vi "Comparing Different Hierarchical Linkage.vi"() -> ()   [LabVIEW 2020]
doc: "This example shows characteristics of different linkage methods for hierarchical clustering on datasets that are “interesting” but still in 2D.\n\nThe main observations to make are :\n\n - single linkage is fast, and can perform well on non-globular data, but it performs poorly in the presence of noise.\n\n- average and complete linkage perform well on cleanly separated globular clusters, but have mixed results otherwise.\n\n- Ward is the most effective method for noisy data.\n\nWhile these examples give some intuition about the algorithms, this intuition might not apply to very high dimensional data."
uses:
  Model/Unsupervised/Cluster/AgglomerativeClustering/controls/agglomerative_clustering_params.ctl
  PLAIYDISPLAY/Display/Classification/2D/Predicted/Controls/PredictedParameter.ctl
  PLAIYDISPLAY/Display/_Controls/Style.ctl
  <vilib>/Analysis/baseanly.llb/Real A x B.vi
  Model/Unsupervised/Cluster/AgglomerativeClustering/AgglomerativeClustering.lvclass
  C:/Users/cipop/TDF Dropbox/2_Technologies de France/1 - Services et Etudes/PLAIY/2 - DEV/PLAIYLAB/code/Model/Model.lvclass
  Preproc/Objet/6 - Datasets Transformation/6.3 - Processing Data/StandardScaler/StandardScaler.vi
  Model/Unsupervised/Cluster/AgglomerativeClustering/AgglomerativeClustering.vi
  <vilib>/Analysis/Matrix/Numeric/Conversions/Array To Matrix - RA2.vi
  <vilib>/Analysis/Matrix/Numeric/Conversions/Matrix To Array - RM.vi
  Preproc/Objet/6 - Datasets Transformation/6.3 - Processing Data/StandardScaler/StandardScaler.lvclass
  <vilib>/Analysis/Matrix/NI_Matrix.lvlib
  <vilib>/Analysis/NI_AALBase.lvlib
panel:
  out "X_aniso":dbl[][](array[numeric])
  in  "error in":errorcluster
  out "error out":errorcluster
  out "Plot 24":cluster{"X":dbl[], "Y":dbl[]}[](graph) caption="Ward Linkage"
  out "no_structure":dbl[][](array[numeric])
  out "Plot 23":cluster{"X":dbl[], "Y":dbl[]}[](graph) caption="Complete Linkage"
  out "Plot 22":cluster{"X":dbl[], "Y":dbl[]}[](graph) caption="Average Linkage"
  out "Plot 21":cluster{"X":dbl[], "Y":dbl[]}[](graph) caption="Single Linkage"
  out "Plot 20":cluster{"X":dbl[], "Y":dbl[]}[](graph) caption="Ward Linkage"
  out "varied":dbl[][](array[numeric])
  out "Plot 19":cluster{"X":dbl[], "Y":dbl[]}[](graph) caption="Complete Linkage"
  out "Plot 18":cluster{"X":dbl[], "Y":dbl[]}[](graph) caption="Average Linkage"
  out "Plot 17":cluster{"X":dbl[], "Y":dbl[]}[](graph) caption="Single Linkage"
  out "Plot 16":cluster{"X":dbl[], "Y":dbl[]}[](graph) caption="Ward Linkage"
  out "aniso":dbl[][](array[numeric])
  out "Plot 15":cluster{"X":dbl[], "Y":dbl[]}[](graph) caption="Complete Linkage"
  out "Plot 14":cluster{"X":dbl[], "Y":dbl[]}[](graph) caption="Average Linkage"
  out "Plot 13":cluster{"X":dbl[], "Y":dbl[]}[](graph) caption="Single Linkage"
  out "Plot 12":cluster{"X":dbl[], "Y":dbl[]}[](graph) caption="Ward Linkage"
  out "blobs":dbl[][](array[numeric])
  out "Plot 11":cluster{"X":dbl[], "Y":dbl[]}[](graph) caption="Complete Linkage"
  out "Plot 10":cluster{"X":dbl[], "Y":dbl[]}[](graph) caption="Average Linkage"
  out "Plot 9":cluster{"X":dbl[], "Y":dbl[]}[](graph) caption="Single Linkage"
  out "Plot 8":cluster{"X":dbl[], "Y":dbl[]}[](graph) caption="Ward Linkage"
  out "noisy_moons":dbl[][](array[numeric])
  out "Plot 7":cluster{"X":dbl[], "Y":dbl[]}[](graph) caption="Complete Linkage"
  out "Plot 6":cluster{"X":dbl[], "Y":dbl[]}[](graph) caption="Average Linkage"
  out "Plot 5":cluster{"X":dbl[], "Y":dbl[]}[](graph) caption="Single Linkage"
  out "Plot 4":cluster{"X":dbl[], "Y":dbl[]}[](graph) caption="Single Linkage"
  out "Plot 3":cluster{"X":dbl[], "Y":dbl[]}[](graph) caption="Average Linkage"
  out "Plot 2":cluster{"X":dbl[], "Y":dbl[]}[](graph) caption="Complete Linkage"
  out "noisy_circles":dbl[][](array[numeric])
  out "Plot":cluster{"X":dbl[], "Y":dbl[]}[](graph) caption="Ward Linkage"
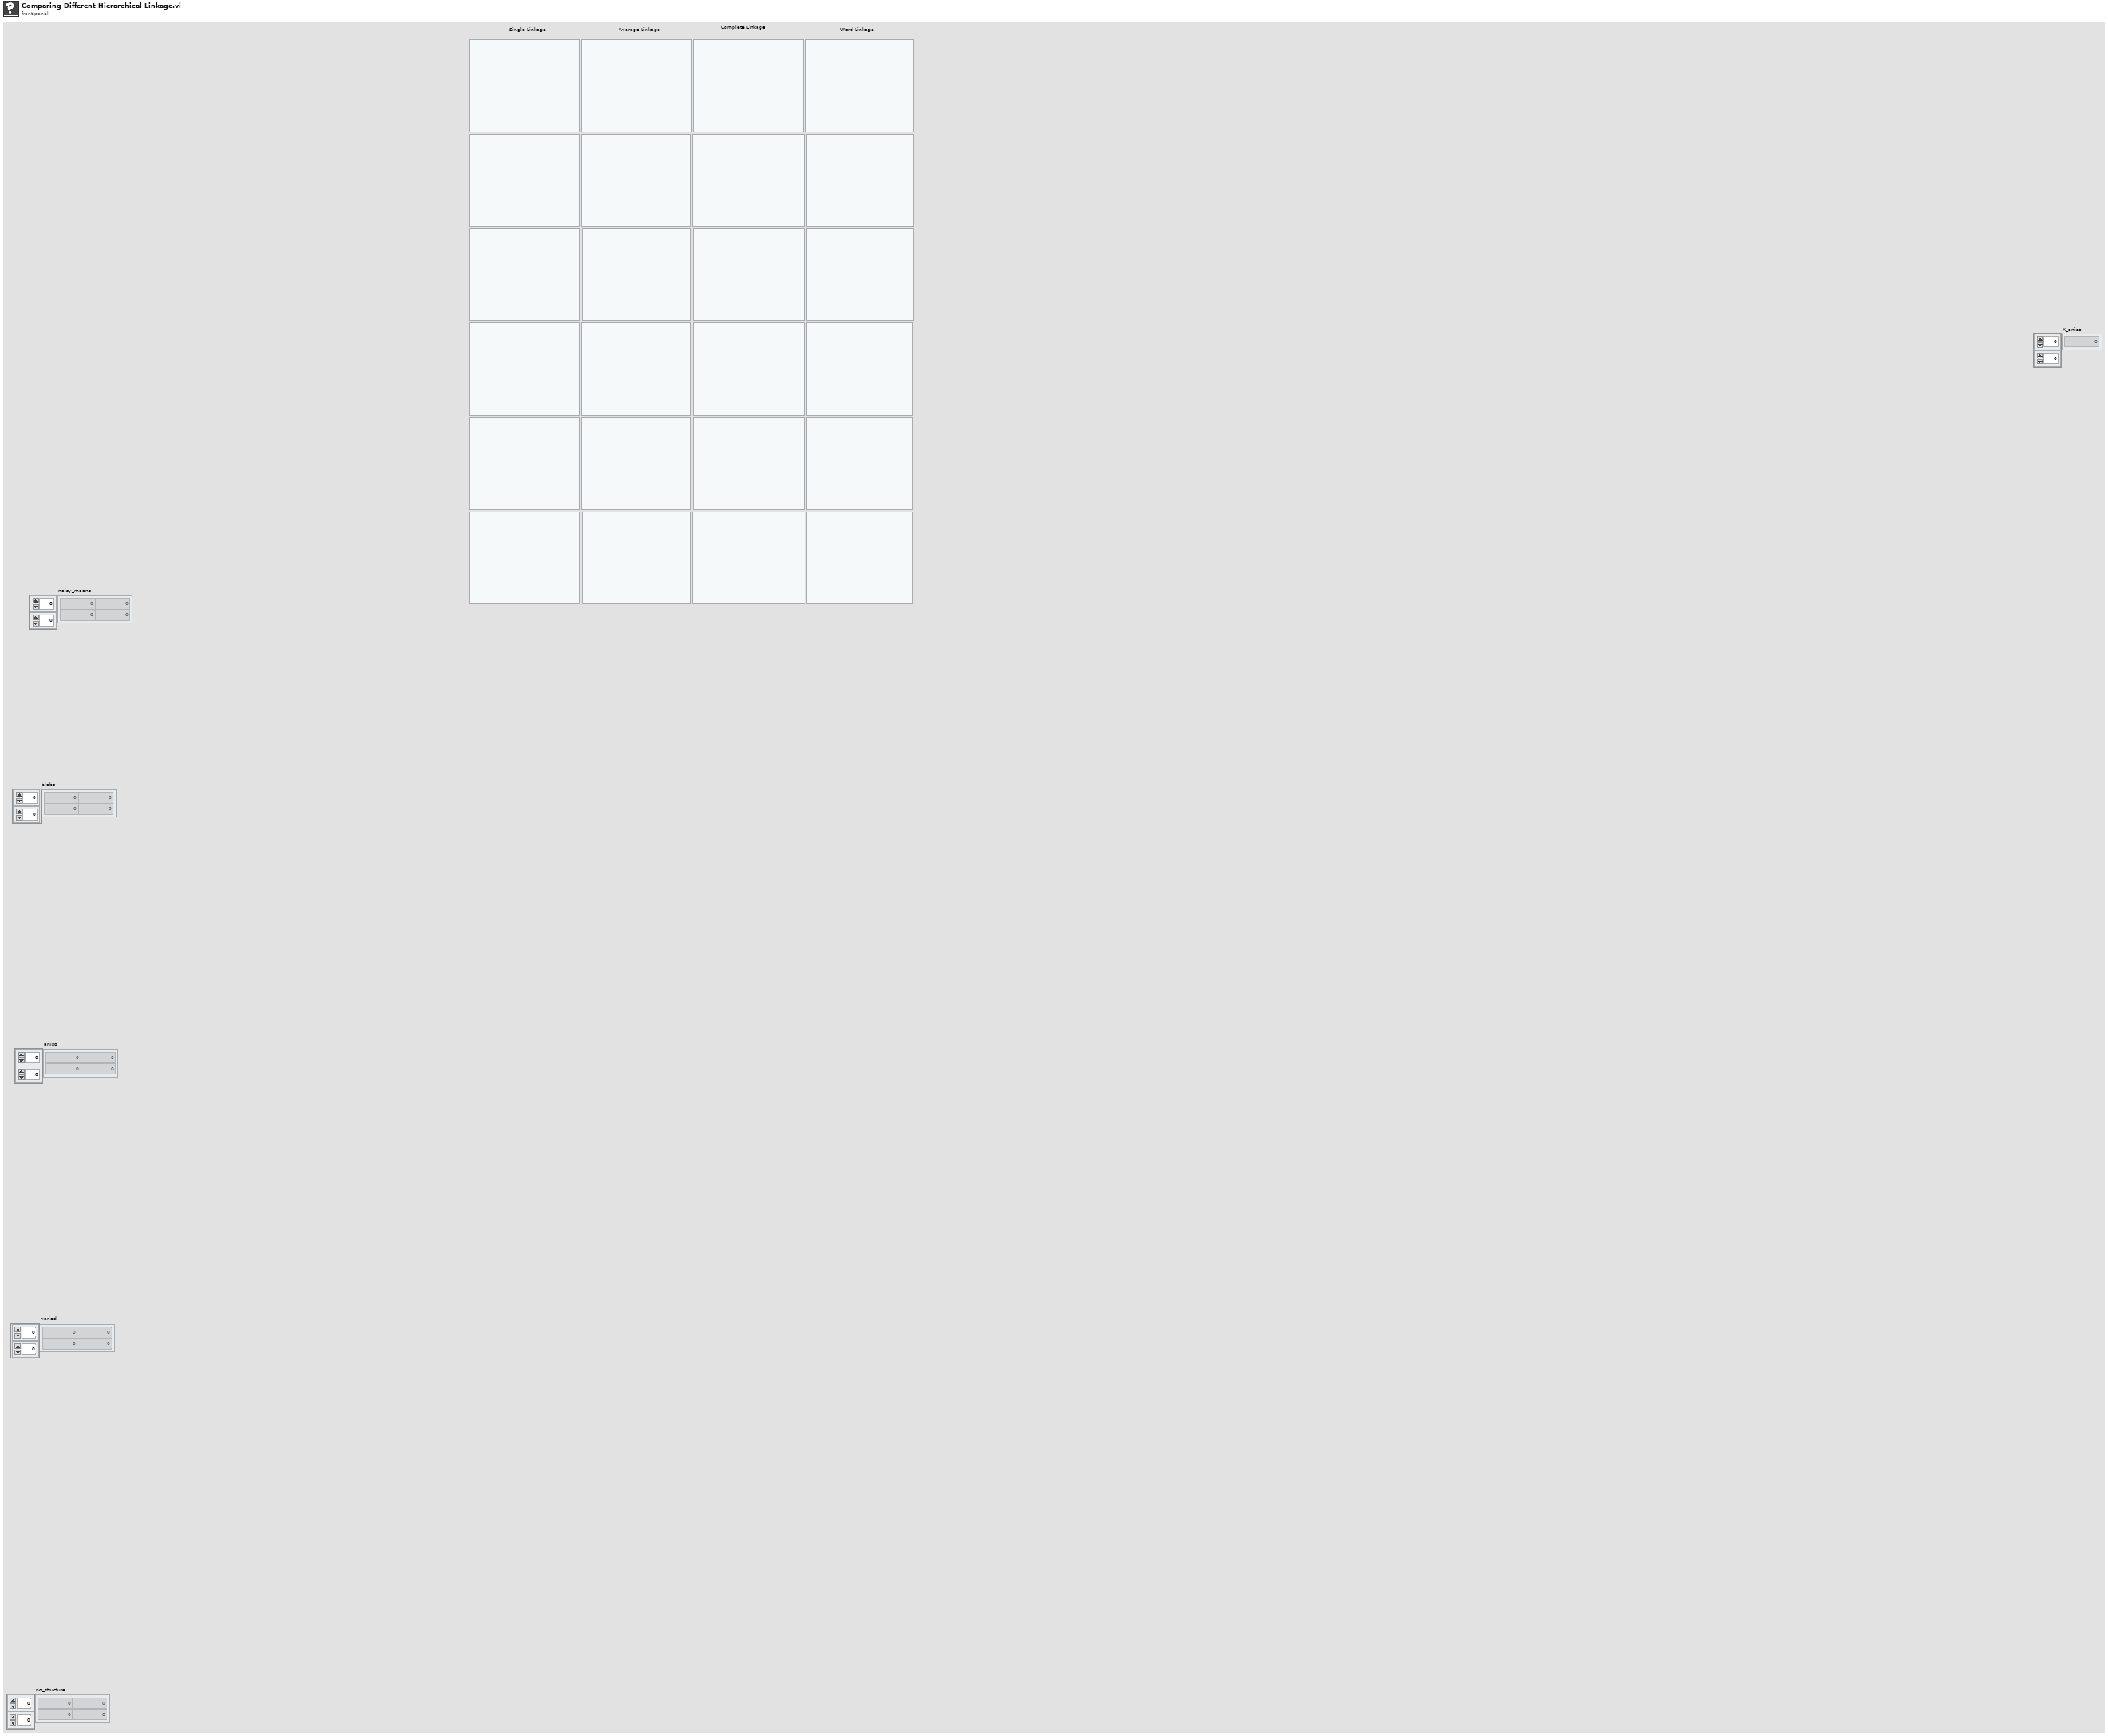
[diagram p1: front panel]
types:
  T1 = enum16{"Numeric Array", "String Array", "Sparse"}
  T2 = cluster{"n_samples":string, "shuffle":bool, "noise":dbl, "random_state":i32, "factor":dbl, "Returns":string}
  T3 = typedef "Style.ctl" = enum16{"Empty circle", "Full circle", "Empty square", "Full square", "Cross"}
  T4 = typedef "PredictedParameter.ctl" = cluster{"Plot":refnum<vi>, "Data":cluster{"X":dbl[][], "Predict":dbl[][]}, "Indexe":cluster{"X":i32, "Y":i32}, "Point Property":cluster{"Style":T3, "Label Color":u32[]}}
  T5 = typedef "agglomerative_clustering_params.ctl" = cluster{"n_clusters":cluster{"n_clusters_type":string, "n_clusters_int":dbl}, "affinity":cluster{"affinity_type":string, "affinity_function":string}, "memory":string, "connectivity":cluster{"connectivity_type":string, "connectivity_list":dbl[][]}, "compute_full_tree":cluster{"compute_full_tree_type":string, "compute_full_tree_bool":bool}, "linkage":string, "distance_threshold":cluster{"distance_threshold_type":string, "distance_threshold_float":dbl}, "compute_distances":bool}
  T6 = cluster{"n_clusters_type":string, "n_clusters_int":dbl}
  T7 = cluster{"n_samples":string, "shuffle":bool, "noise":dbl, "random_state":i32, "Returns":string}
  T8 = cluster{"n_samples":i32[], "n_features":u32, "centers":i32[][], "cluster_std":dbl[], "centermin":dbl, "centermax":dbl, "shuffle":bool, "random_state":i32, "Returns":string}
  T9 = cluster{" 4DArray":cluster{"1":string[][], "2":string[][]}[], " 3DArray":cluster{"Tableau":string[][]}[], "Sparse Matrix 2DArray":string[][], " 2DArray":string[][], " 1DArray":string[]}
  T10 = typedef "agglomerative_clustering_attributes.ctl" = cluster{"n_clusters_":dbl, "labels_":dbl[], "n_leaves_":dbl, "n_connected_components_":dbl, "children_":dbl[][], "distances_":dbl[]}
  T11 = typedef "NI_Matrix.lvlib/RealMatrix.ctl" = dbl[][]
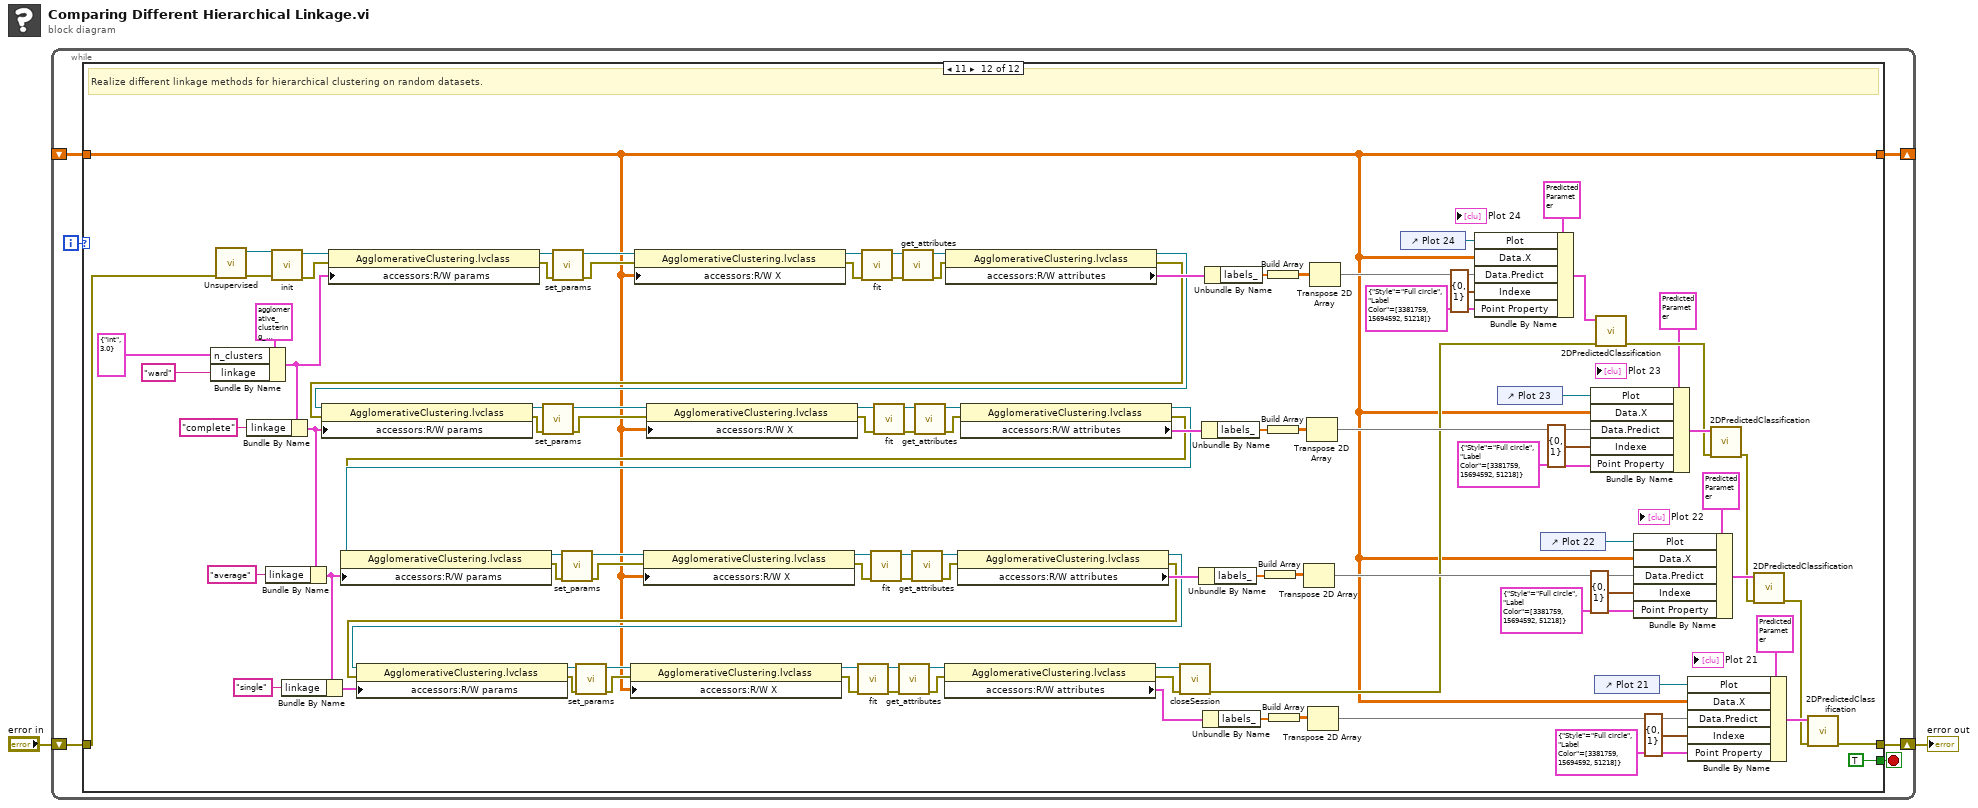
[diagram p0: block diagram]
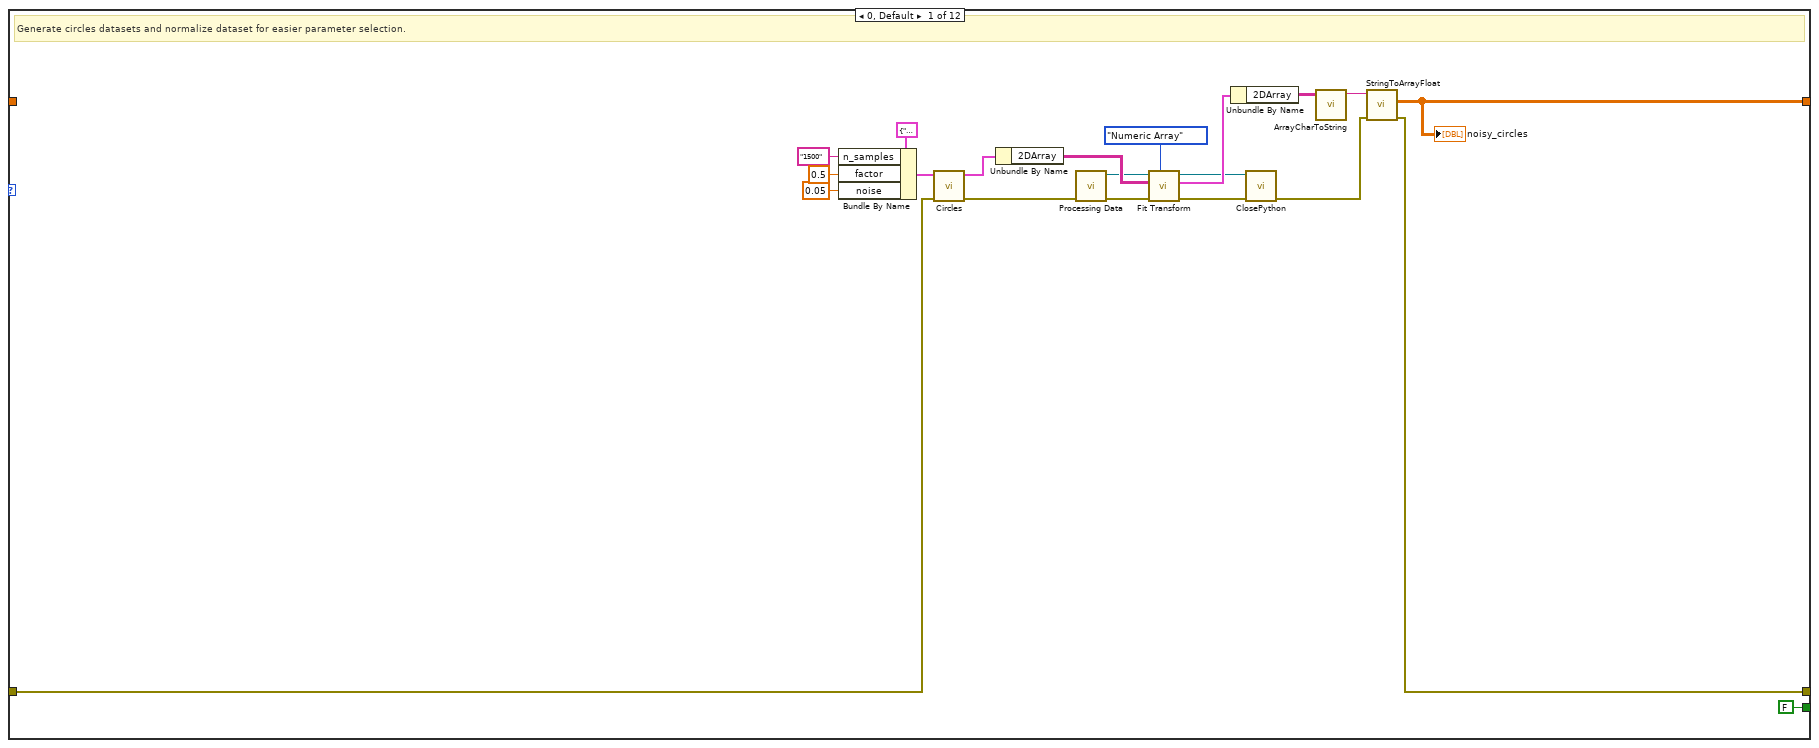
[diagram p2: hidden frame]
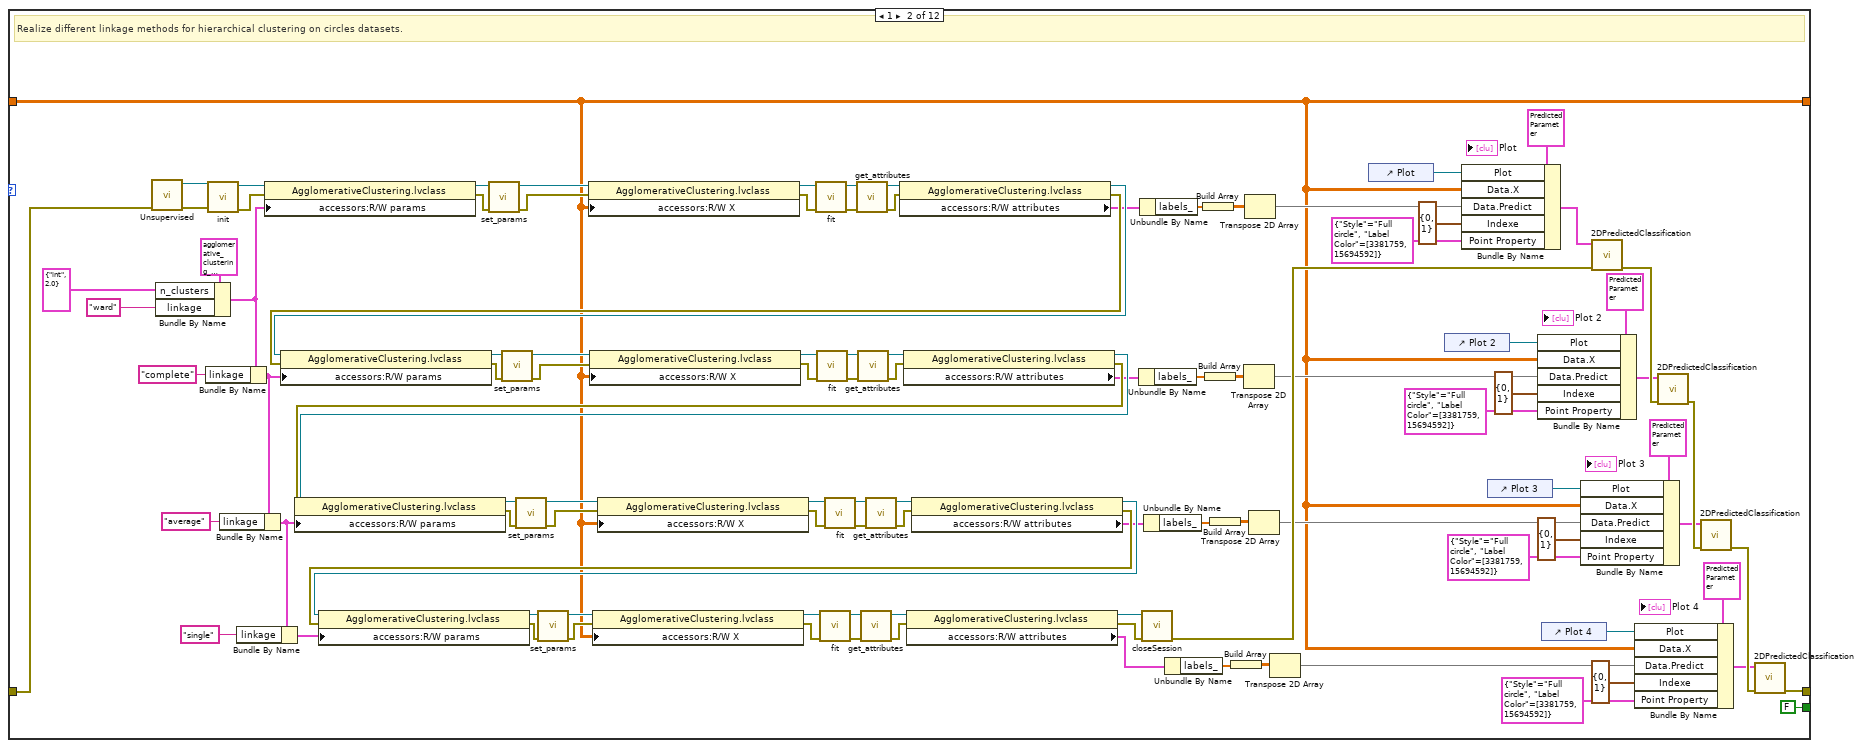
[diagram p3: hidden frame]
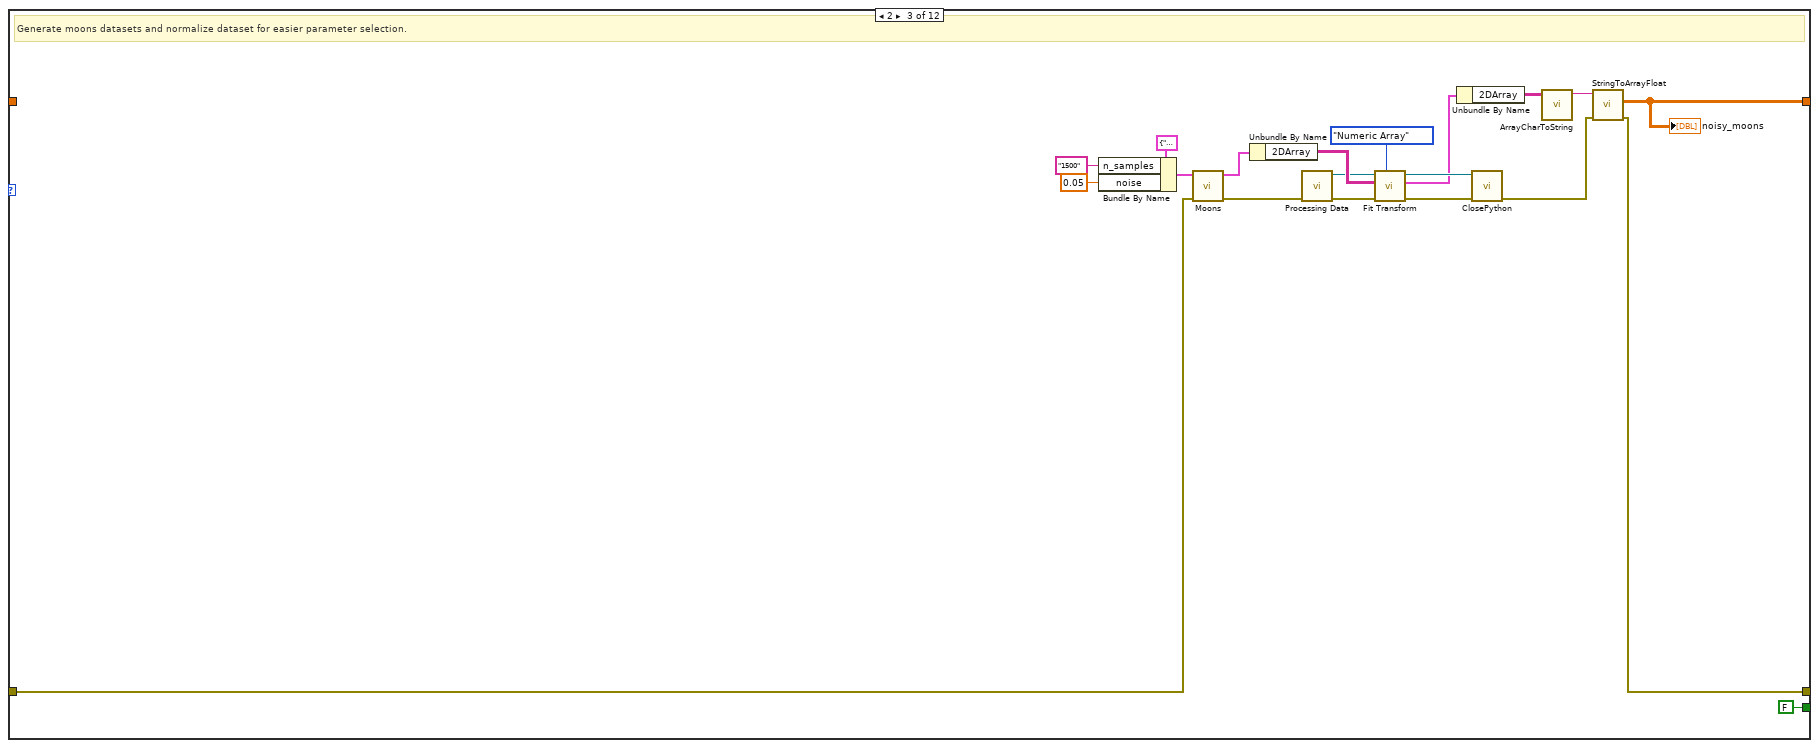
[diagram p4: hidden frame]
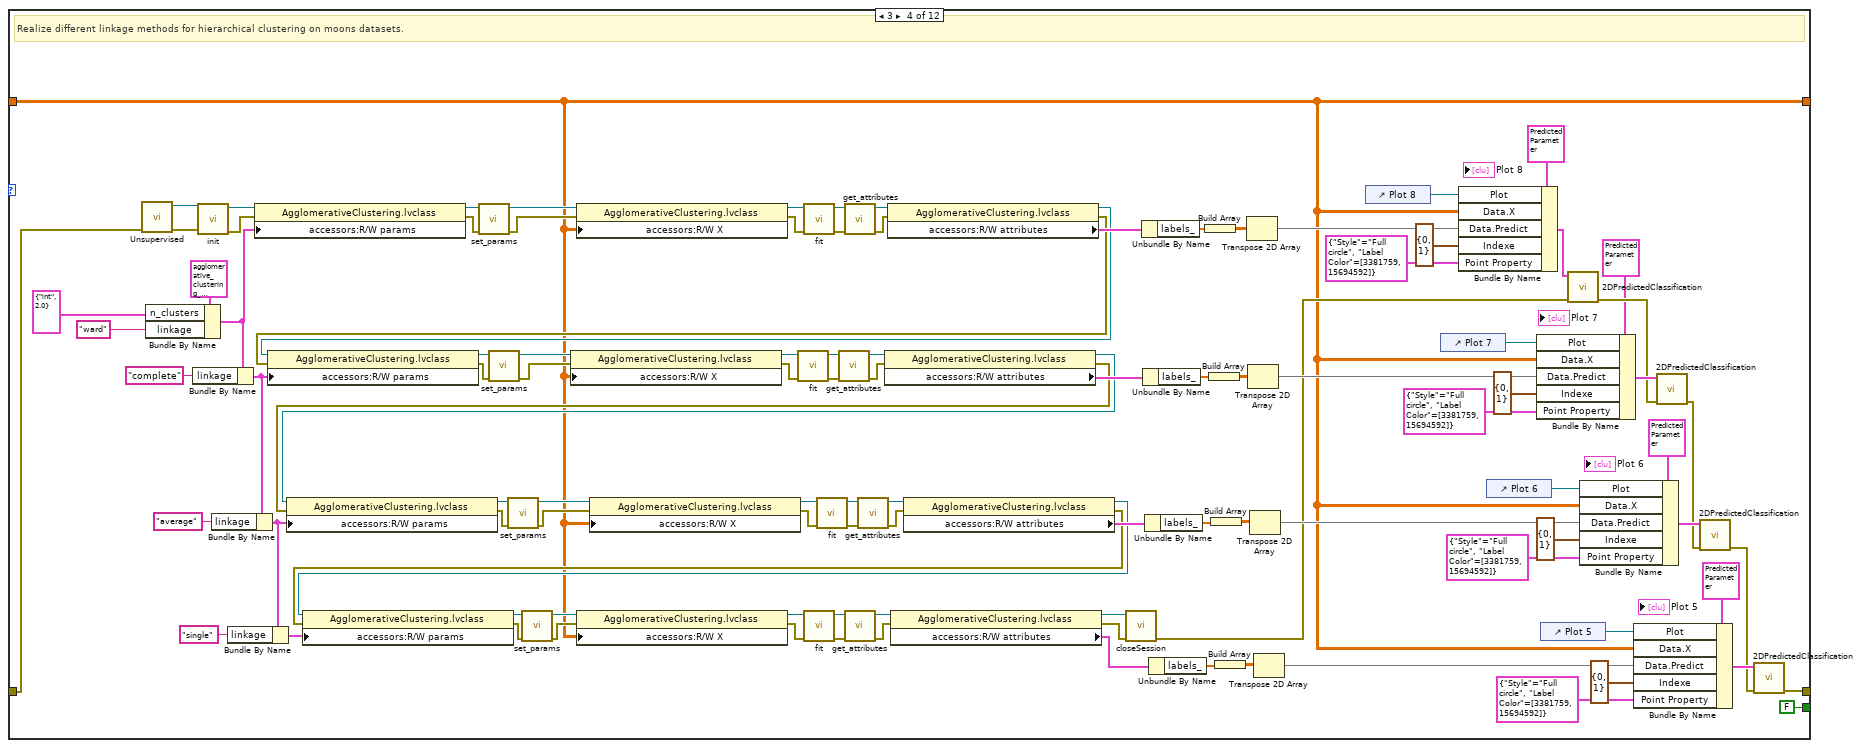
[diagram p5: hidden frame]
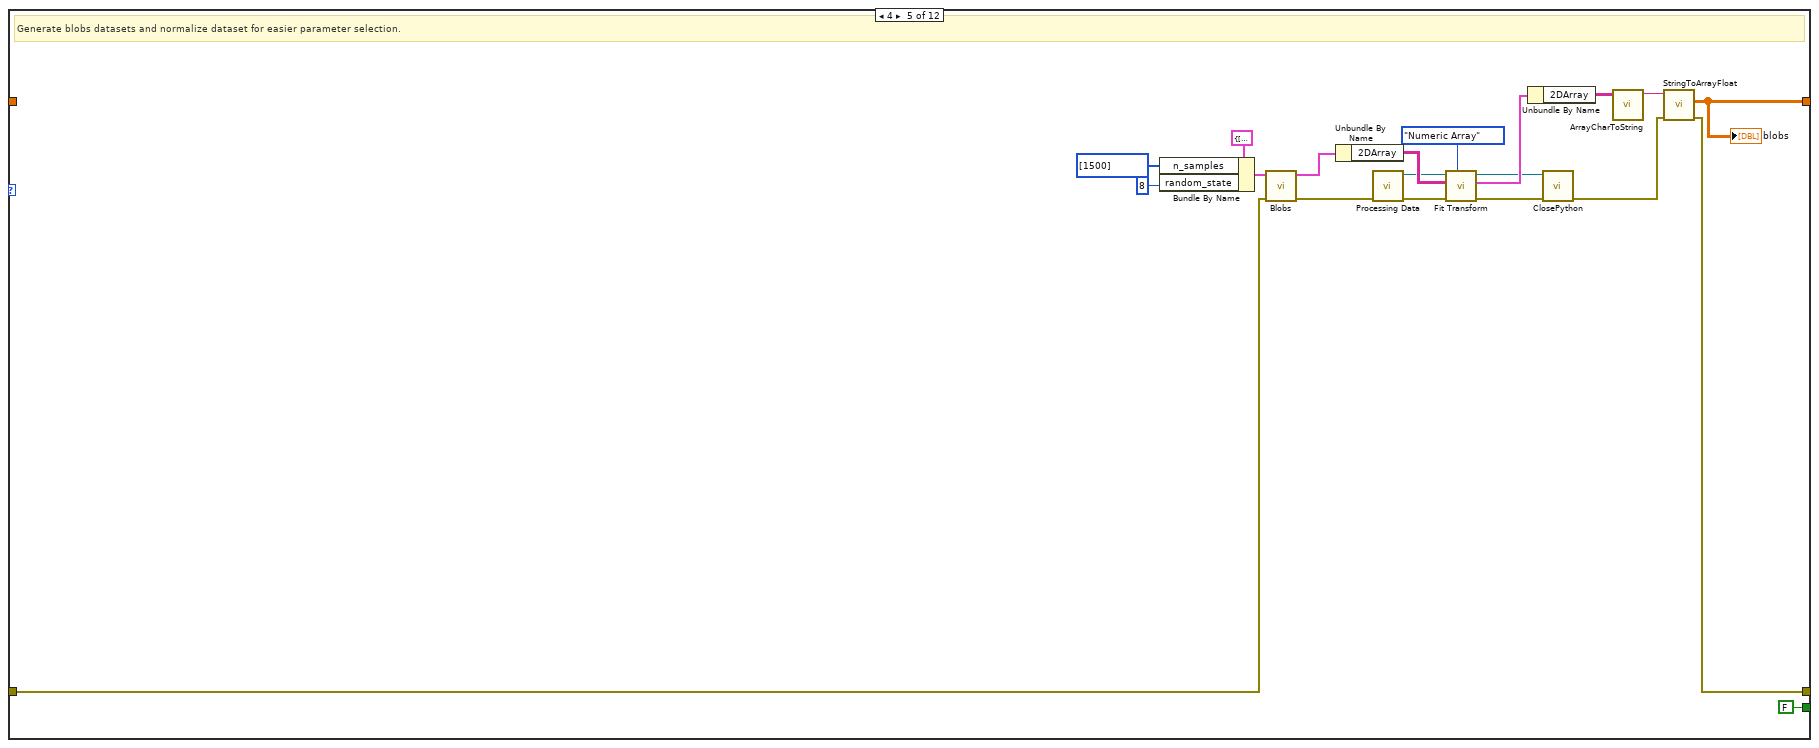
[diagram p6: hidden frame]
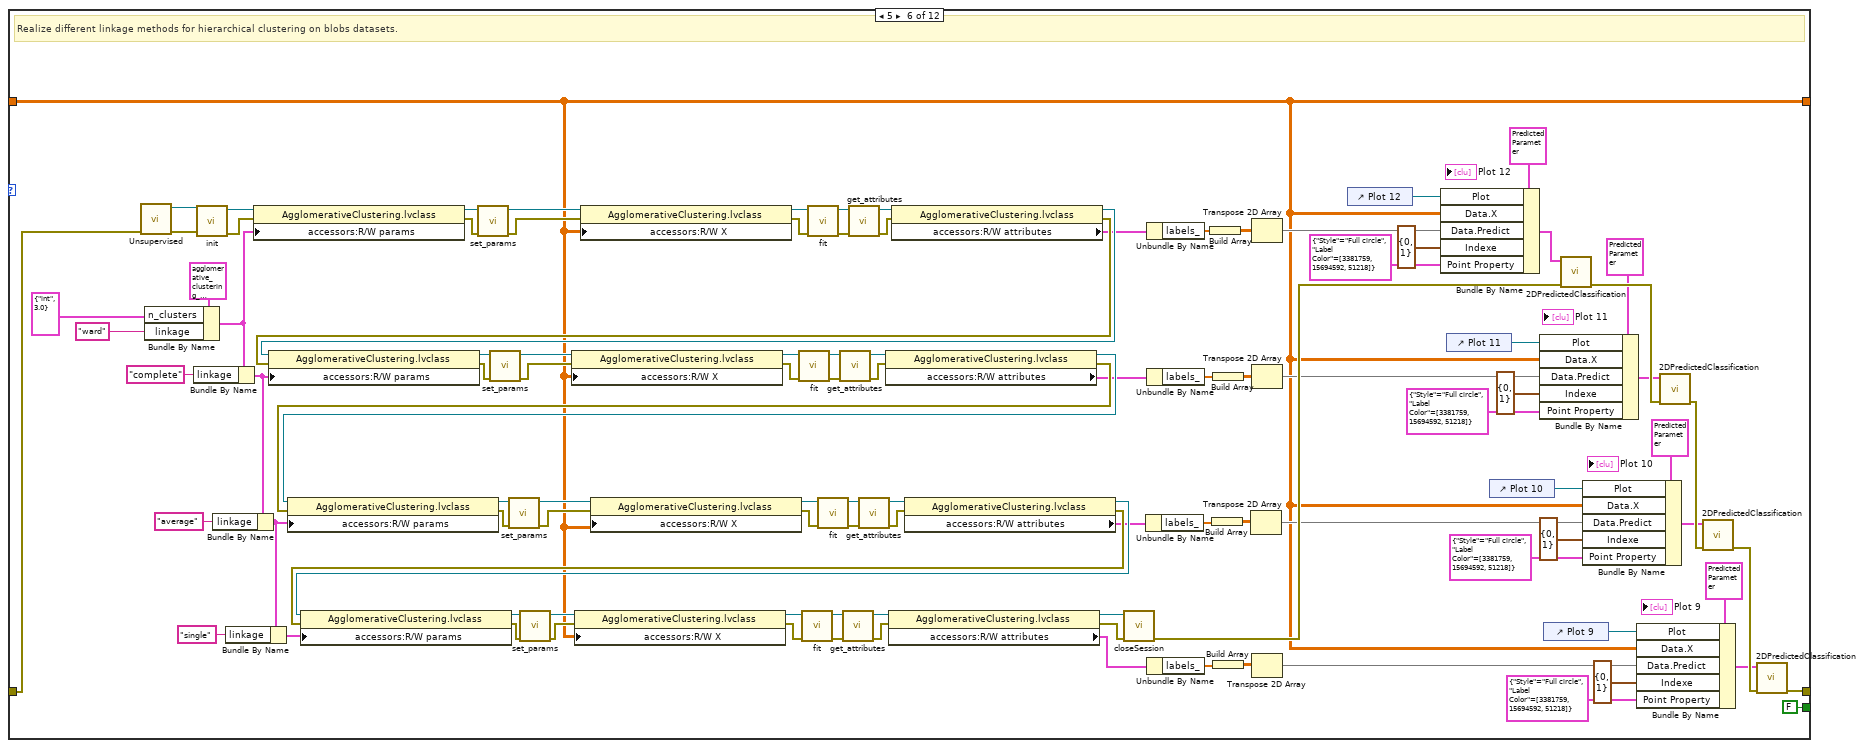
[diagram p7: hidden frame]
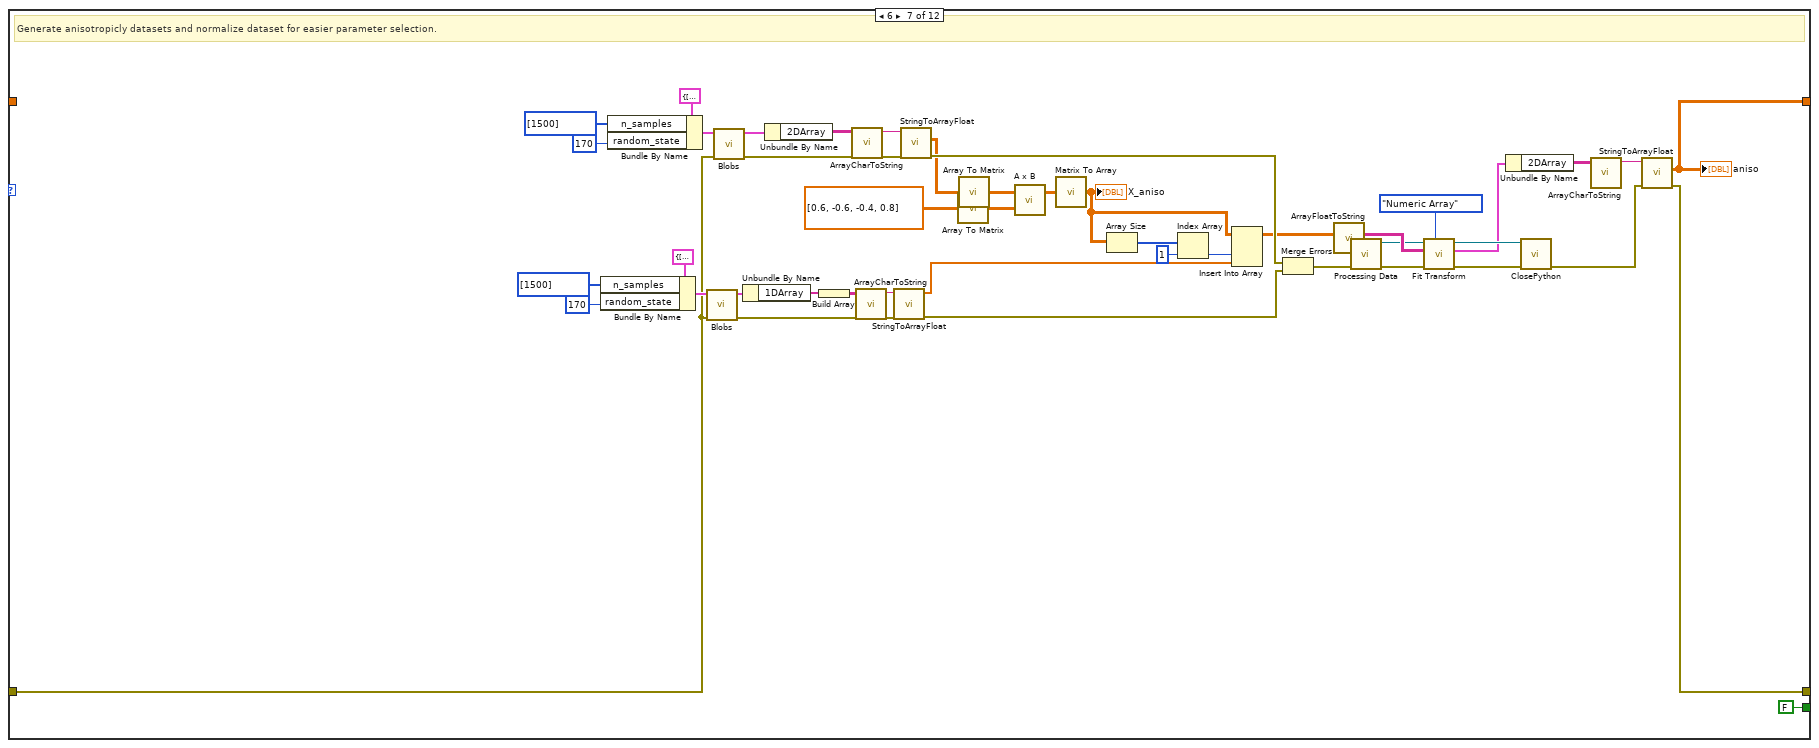
[diagram p8: hidden frame]
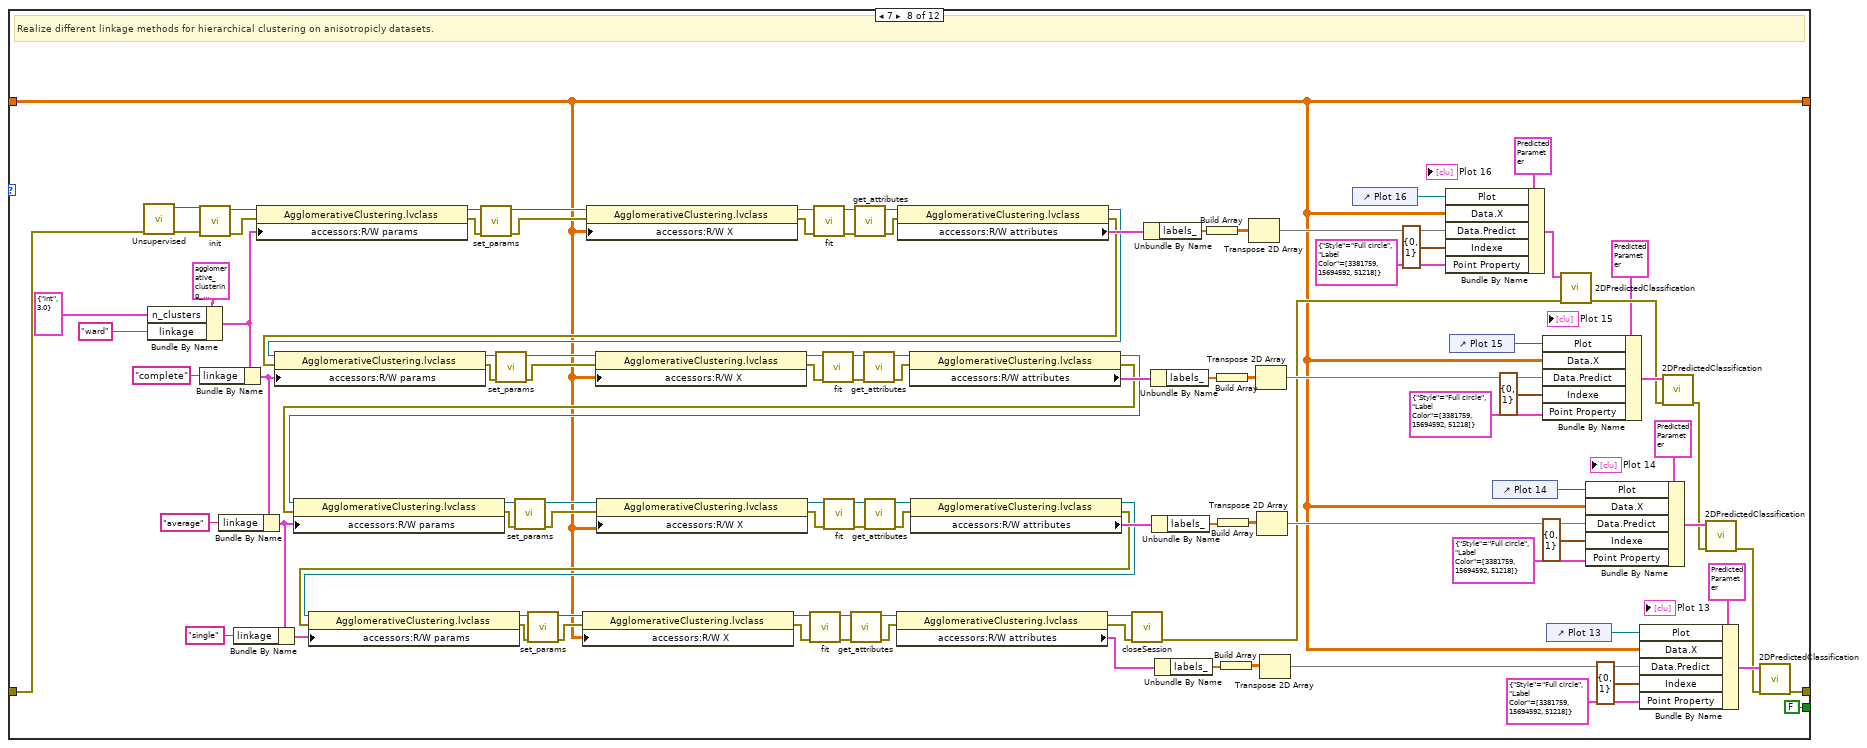
[diagram p9: hidden frame]
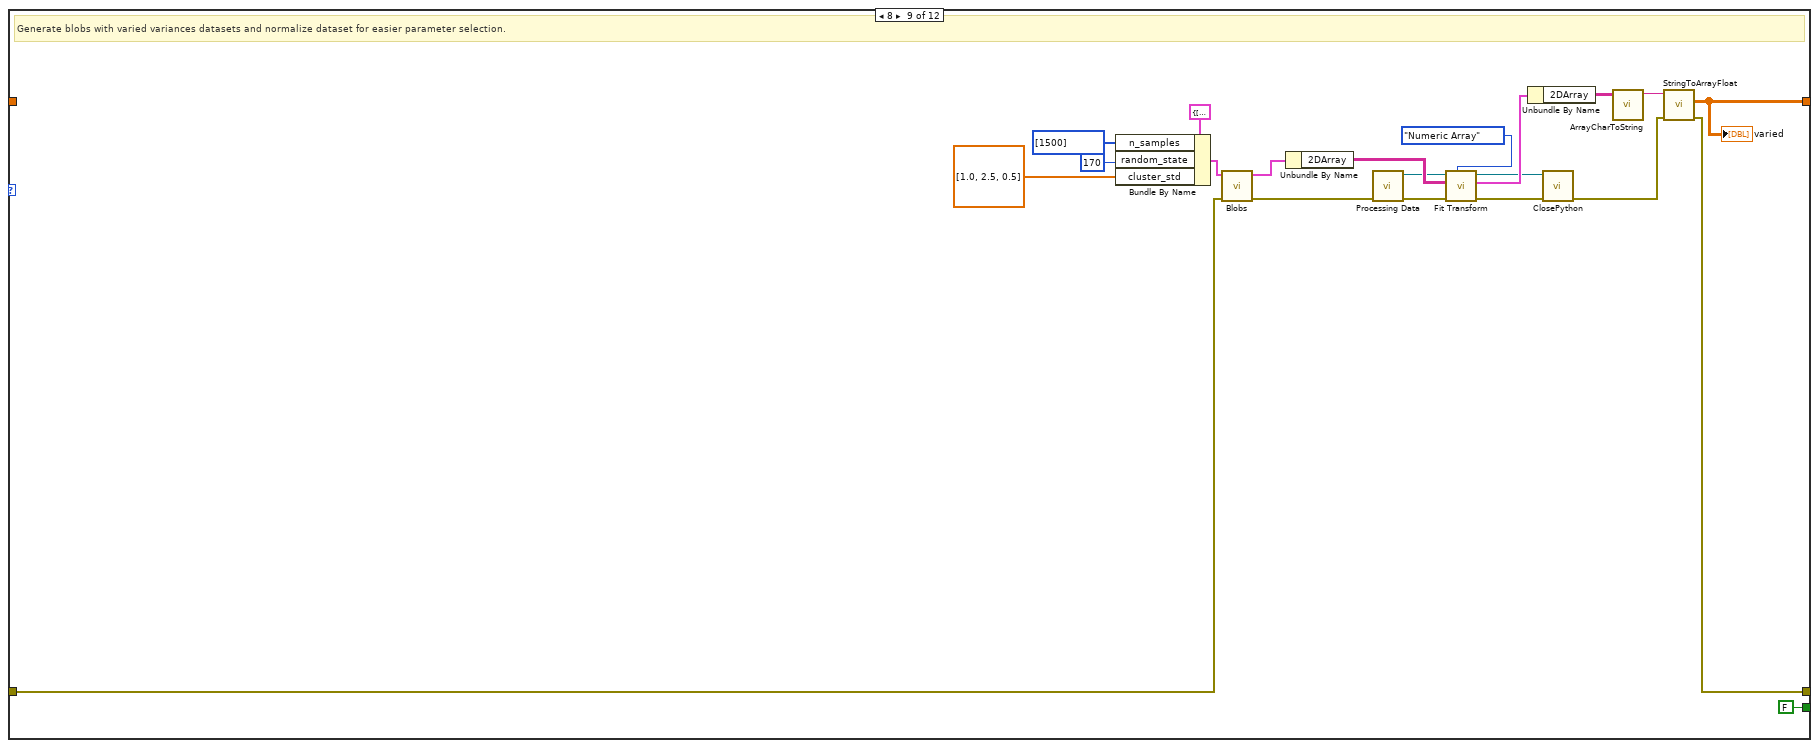
[diagram p10: hidden frame]
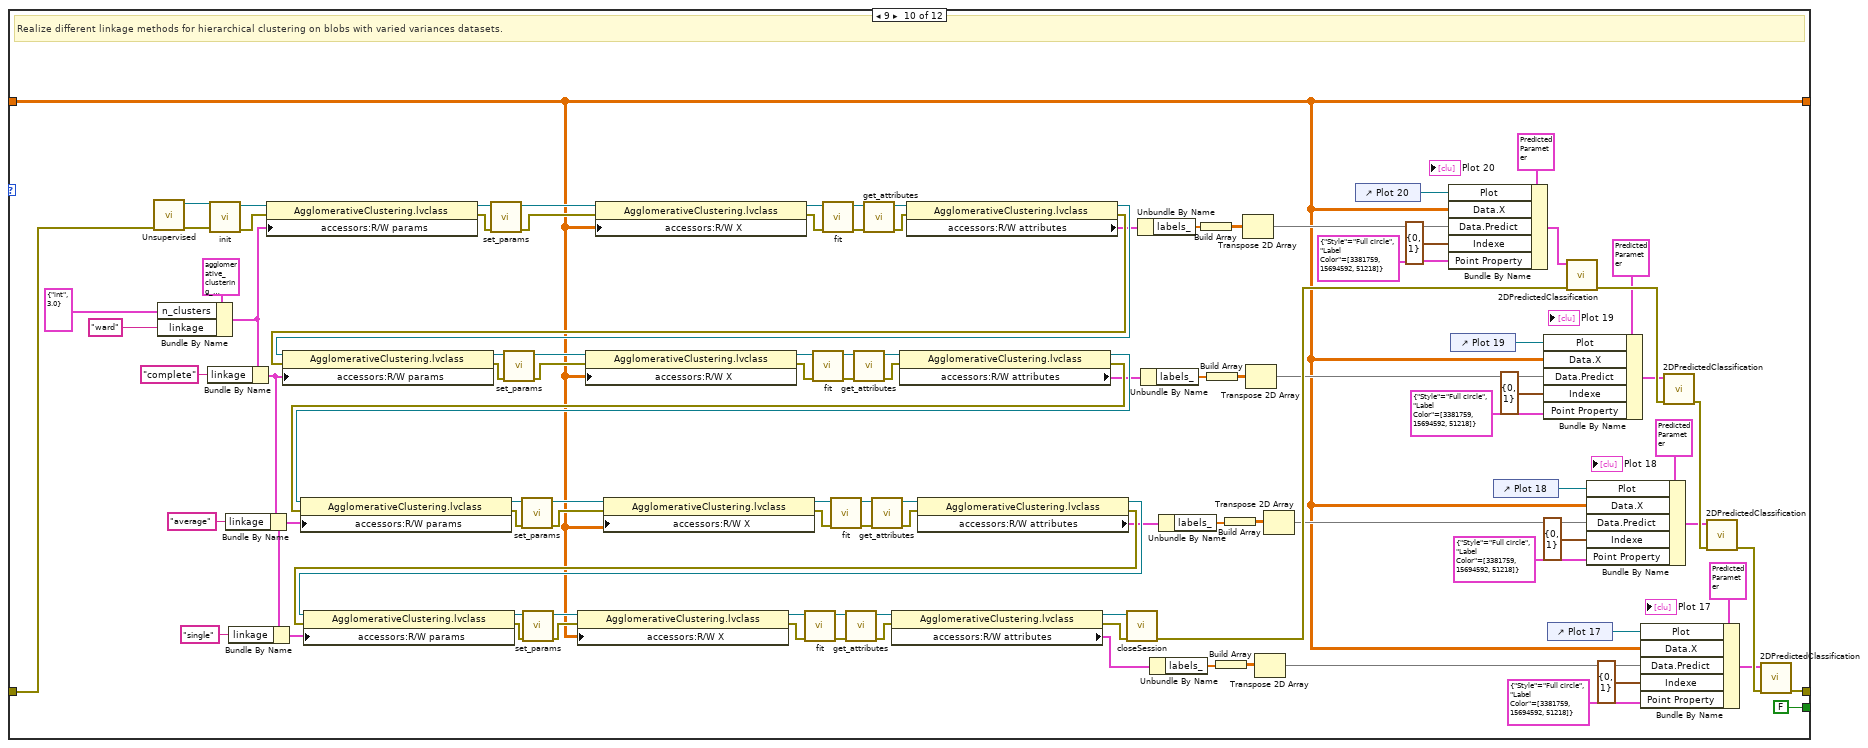
[diagram p11: hidden frame]
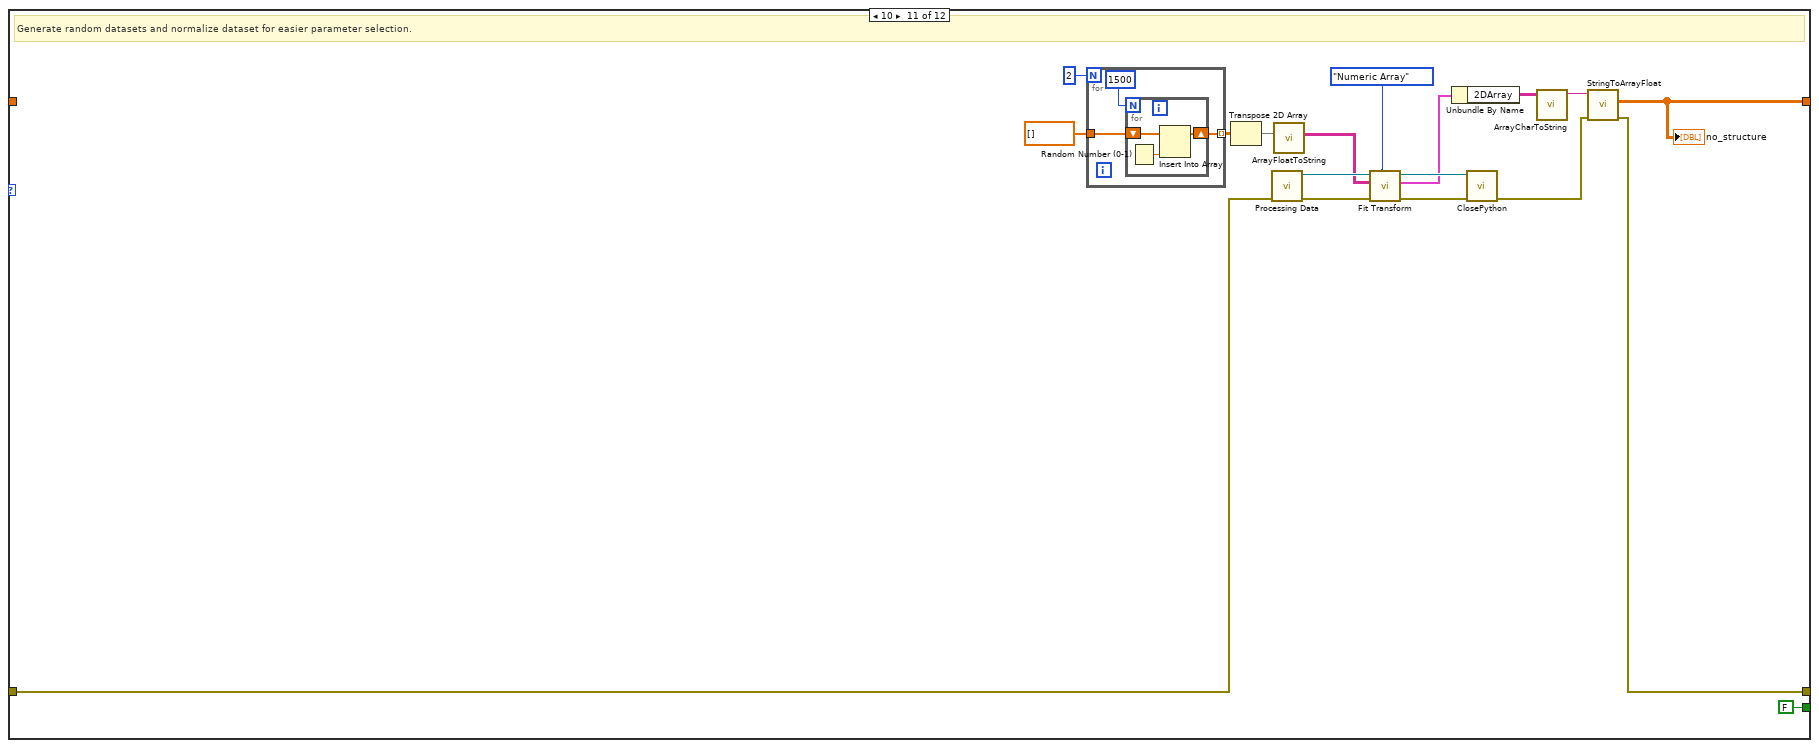
[diagram p12: hidden frame]
diagram:
  n1 = while {
    shift-right: [w5] -> w1
    shift-left: "error in" -> [w6]
    shift-right: [w4] -> _
    shift-left: _ -> [w3]
    i -> [w8]
    stop <- w7 stop-if-true
    n2 = case shown="11" w8 {
      tunnel: [FALSE FALSE FALSE FALSE FALSE FALSE FALSE FALSE FALSE FALSE FALSE TRUE] -> w7
      tunnel: w6 -> [w12 w31 w137 w157 w263 w283 w391 w434 w540 w561 w667 w691]
      tunnel: [w10 w32 w139 w162 w265 w288 w390 w435 w542 w562 w669 w693] -> w5
      tunnel: [w11 w30 w136 w156 w262 w282 w388 w433 w539 w560 w666 w690] -> w4
      tunnel: w3 -> [_ w30 _ w156 _ w282 _ w433 _ w560 _ w690]
      frame 0, Default {
        # "Generate circles datasets and normalize dataset for easier parameter selection."
        n3 = Bundle By Name(cluster=T2 {"n_samples"="100", "shuffle"=TRUE, "noise"=-1.0, "random_state"=-1, "factor"=0.8, "Returns"="X"} ("make_circles"), "n_samples"="1500", "factor"=0.5, "noise"=0.05) -> (w19:T2)
        n4 = call "Circles.vi"("error in (no error)"=w12, "make_circles"=w19) -> ("error out"=w26:errorcluster, "Data"=w18:T9)  [unwired: 8 in]
        n5 = Unbundle By Name(w18) -> ("2DArray"=w24:string[][])
        n6 = call-poly "Processing Data.vi"("error in (no error)"=w26) -> ("error out"=w21:errorcluster, "StandardScaler.lvclass"=w20:refnum<class "StandardScaler.lvclass">)  [unwired: 9 in]
        n7 = call-dynamic "Fit Transform.vi"("Type X"=T1."Numeric Array", "error in (no error)"=w21, "X"=w24, "StandardScaler.lvclass"=w20) -> ("error out"=w23:errorcluster, "Data"=w25:T9, "StandardScaler.lvclass"=w22:refnum<class "StandardScaler.lvclass">)  [unwired: 5 in]
        n8 = Unbundle By Name(w25) -> ("2DArray"=w28:string[][])
        n9 = call-dynamic "ClosePython.vi"("error in (no error)"=w23, "Scikit-learn en entrée"=w22) -> ("error out"=w29:errorcluster)  [unwired: 8 in, 1 out]
        n10 = call "ArrayCharToString.vi"("TAB"=w28) -> ("Instruction"=w27:string)  [unwired: 10 in]
        n11 = call "StringToArrayFloat.vi"("entrée d'erreur (pas d'erreur)"=w29, "Return value"=w27) -> ("error IO"=w10:errorcluster, "2DArray"=w11:dbl[][])  [unwired: 7 in, 1 out]
        "noisy_circles" <- w11
      }
      frame 1 {
        # "Realize different linkage methods for hierarchical clustering on circles datasets."
        n12 = call-poly "Unsupervised.vi"("error in"=w31) -> ("error out"=w57:errorcluster, "out"=w56:refnum<class "AgglomerativeClustering.lvclass">)  [unwired: 9 in]
        n13 = Bundle By Name(cluster=T5 {"n_clusters"={"n_clusters_type"="int", "n_clusters_int"=0.0}, "affinity"={"affinity_type"="euclidean", "affinity_function"="metric_function"}, "memory"="", "connectivity"={"connectivity_type"="None", "connectivity_list"=[]}, "compute_full_tree"={"compute_full_tree_type"="auto", "compute_full_tree_bool"=FALSE}, "linkage"="ward", "distance_threshold"={"distance_threshold_type"="None", "distance_threshold_float"=0.0}, "compute_distances"=FALSE} ("output cluster"), "n_clusters"=T6 {"n_clusters_type"="int", "n_clusters_int"=2.0}, "linkage"="ward") -> (w81:T5)
        n14 = Bundle By Name(cluster=w81, "linkage"="complete") -> (w96:T5)
        n15 = call-dynamic "init.vi"("error in (no error)"=w57, "Model en entrée"=w56) -> ("error out"=w58:errorcluster, "Model en sortie"=w52:refnum<class "AgglomerativeClustering.lvclass">)  [unwired: 8 in]
        n16 = Bundle By Name(cluster=w96, "linkage"="average") -> (w114:T5)
        n17 = Bundle By Name(cluster=w114, "linkage"="single") -> (w112:T5)
        n18 = property class="AgglomerativeClustering.lvclass"(reference=w52, error in=w58, "accessors:R/W params"=w81) -> (reference out=w53:refnum<class "AgglomerativeClustering.lvclass">, error out=w59:errorcluster)
        n19 = call-dynamic "set_params.vi"("error in (no error)"=w59, "AgglomerativeClustering.lvclass 2"=w53) -> ("error out"=w60:errorcluster, "AgglomerativeClustering.lvclass"=w54:refnum<class "AgglomerativeClustering.lvclass">)  [unwired: 8 in]
        n20 = property class="AgglomerativeClustering.lvclass"(reference=w54, error in=w60, "accessors:R/W X"=w30) -> (reference out=w51:refnum<class "AgglomerativeClustering.lvclass">, error out=w61:errorcluster)
        n21 = call-dynamic "fit.vi"("error in (no error)"=w61, "AgglomerativeClustering.lvclass 2"=w51) -> ("error out"=w62:errorcluster, "AgglomerativeClustering.lvclass"=w55:refnum<class "AgglomerativeClustering.lvclass">)  [unwired: 8 in]
        n22 = call-dynamic "get_attributes.vi"("error in (no error)"=w62, "AgglomerativeClustering.lvclass 2"=w55) -> ("error out"=w68:errorcluster, "AgglomerativeClustering.lvclass"=w67:refnum<class "AgglomerativeClustering.lvclass">)  [unwired: 8 in]
        n23 = property class="AgglomerativeClustering.lvclass"(reference=w67, error in=w68) -> (reference out=w82:refnum<class "AgglomerativeClustering.lvclass">, error out=w83:errorcluster, "accessors:R/W attributes"=w63:T10)
        n24 = property class="AgglomerativeClustering.lvclass"(reference=w82, error in=w83, "accessors:R/W params"=w96) -> (reference out=w79:refnum<class "AgglomerativeClustering.lvclass">, error out=w76:errorcluster)
        n25 = call-dynamic "set_params.vi"("error in (no error)"=w76, "AgglomerativeClustering.lvclass 2"=w79) -> ("error out"=w75:errorcluster, "AgglomerativeClustering.lvclass"=w78:refnum<class "AgglomerativeClustering.lvclass">)  [unwired: 8 in]
        n26 = property class="AgglomerativeClustering.lvclass"(reference=w78, error in=w75, "accessors:R/W X"=w30) -> (reference out=w80:refnum<class "AgglomerativeClustering.lvclass">, error out=w74:errorcluster)
        n27 = call-dynamic "fit.vi"("error in (no error)"=w74, "AgglomerativeClustering.lvclass 2"=w80) -> ("error out"=w73:errorcluster, "AgglomerativeClustering.lvclass"=w77:refnum<class "AgglomerativeClustering.lvclass">)  [unwired: 8 in]
        n28 = call-dynamic "get_attributes.vi"("error in (no error)"=w73, "AgglomerativeClustering.lvclass 2"=w77) -> ("error out"=w71:errorcluster, "AgglomerativeClustering.lvclass"=w72:refnum<class "AgglomerativeClustering.lvclass">)  [unwired: 8 in]
        n29 = property class="AgglomerativeClustering.lvclass"(reference=w72, error in=w71) -> (reference out=w97:refnum<class "AgglomerativeClustering.lvclass">, error out=w98:errorcluster, "accessors:R/W attributes"=w86:T10)
        n30 = property class="AgglomerativeClustering.lvclass"(reference=w97, error in=w98, "accessors:R/W params"=w114) -> (reference out=w99:refnum<class "AgglomerativeClustering.lvclass">, error out=w91:errorcluster)
        n31 = call-dynamic "set_params.vi"("error in (no error)"=w91, "AgglomerativeClustering.lvclass 2"=w99) -> ("error out"=w92:errorcluster, "AgglomerativeClustering.lvclass"=w100:refnum<class "AgglomerativeClustering.lvclass">)  [unwired: 8 in]
        n32 = property class="AgglomerativeClustering.lvclass"(reference=w100, error in=w92, "accessors:R/W X"=w30) -> (reference out=w117:refnum<class "AgglomerativeClustering.lvclass">, error out=w93:errorcluster)
        n33 = call-dynamic "fit.vi"("error in (no error)"=w93, "AgglomerativeClustering.lvclass 2"=w117) -> ("error out"=w94:errorcluster, "AgglomerativeClustering.lvclass"=w118:refnum<class "AgglomerativeClustering.lvclass">)  [unwired: 8 in]
        n34 = call-dynamic "get_attributes.vi"("error in (no error)"=w94, "AgglomerativeClustering.lvclass 2"=w118) -> ("error out"=w95:errorcluster, "AgglomerativeClustering.lvclass"=w119:refnum<class "AgglomerativeClustering.lvclass">)  [unwired: 8 in]
        n35 = property class="AgglomerativeClustering.lvclass"(reference=w119, error in=w95) -> (reference out=w120:refnum<class "AgglomerativeClustering.lvclass">, error out=w121:errorcluster, "accessors:R/W attributes"=w101:T10)
        n36 = property class="AgglomerativeClustering.lvclass"(reference=w120, error in=w121, "accessors:R/W params"=w112) -> (reference out=w115:refnum<class "AgglomerativeClustering.lvclass">, error out=w111:errorcluster)
        n37 = call-dynamic "set_params.vi"("error in (no error)"=w111, "AgglomerativeClustering.lvclass 2"=w115) -> ("error out"=w127:errorcluster, "AgglomerativeClustering.lvclass"=w126:refnum<class "AgglomerativeClustering.lvclass">)  [unwired: 8 in]
        n38 = property class="AgglomerativeClustering.lvclass"(reference=w126, error in=w127, "accessors:R/W X"=w30) -> (reference out=w125:refnum<class "AgglomerativeClustering.lvclass">, error out=w110:errorcluster)
        n39 = call-dynamic "fit.vi"("error in (no error)"=w110, "AgglomerativeClustering.lvclass 2"=w125) -> ("error out"=w109:errorcluster, "AgglomerativeClustering.lvclass"=w124:refnum<class "AgglomerativeClustering.lvclass">)  [unwired: 8 in]
        n40 = call-dynamic "get_attributes.vi"("error in (no error)"=w109, "AgglomerativeClustering.lvclass 2"=w124) -> ("error out"=w108:errorcluster, "AgglomerativeClustering.lvclass"=w123:refnum<class "AgglomerativeClustering.lvclass">)  [unwired: 8 in]
        n41 = property class="AgglomerativeClustering.lvclass"(reference=w123, error in=w108) -> (reference out=w122:refnum<class "AgglomerativeClustering.lvclass">, error out=w113:errorcluster, "accessors:R/W attributes"=w130:T10)
        n42 = Unbundle By Name(w86) -> ("labels_"=w85:dbl[])
        n43 = Unbundle By Name(w63) -> ("labels_"=w66:dbl[])
        n44 = call-dynamic "closeSession.vi"("error in"=w113, "Python en entrée"=w122) -> ("error out"=w116:errorcluster)  [unwired: 8 in, 1 out]
        n45 = Unbundle By Name(w101) -> ("labels_"=w103:dbl[])
        n46 = Unbundle By Name(w130) -> ("labels_"=w128:dbl[])
        n47 = Build Array(w66) -> (w69:dbl[][])
        n48 = Build Array(w85) -> (w84:dbl[][])
        n49 = Build Array(w103) -> (w102:dbl[][])
        n50 = Build Array(w128) -> (w129:dbl[][])
        n51 = Transpose 2D Array(2D array=w84) -> (transposed array=w90:dbl[][])
        n52 = Transpose 2D Array(2D array=w69) -> (transposed array=w70:dbl[][])
        n53 = Transpose 2D Array(2D array=w102) -> (transposed array=w107:dbl[][])
        n54 = Transpose 2D Array(2D array=w129) -> (transposed array=w134:dbl[][])
        n55 = control-ref of="Plot"() -> (w64:refnum<vi>)
        n56 = control-ref of="Plot 2"() -> (w88:refnum<vi>)
        n57 = Bundle By Name(cluster=T4 {"Plot"=refnum, "Data"={"X"=[], "Predict"=[]}, "Indexe"={"X"=0, "Y"=1}, "Point Property"={"Style"=enum."Full circle", "Label Color"=[8978528, 4367871, 1985280]}} ("Parameters"), "Plot"=w64, "Data.X"=w30, "Data.Predict"=w70, "Indexe"=cluster{"X":i32, "Y":i32} {"X"=0, "Y"=1}, "Point Property"=cluster{"Style":T3, "Label Color":u32[]} {"Style"=enum."Full circle", "Label Color"=[3381759, 15694592]}) -> (w65:T4)
        n58 = control-ref of="Plot 3"() -> (w104:refnum<vi>)
        n59 = Bundle By Name(cluster=T4 {"Plot"=refnum, "Data"={"X"=[], "Predict"=[]}, "Indexe"={"X"=0, "Y"=1}, "Point Property"={"Style"=enum."Full circle", "Label Color"=[8978528, 4367871, 1985280]}} ("Parameters"), "Plot"=w88, "Data.X"=w30, "Data.Predict"=w90, "Indexe"=cluster{"X":i32, "Y":i32} {"X"=0, "Y"=1}, "Point Property"=cluster{"Style":T3, "Label Color":u32[]} {"Style"=enum."Full circle", "Label Color"=[3381759, 15694592]}) -> (w87:T4)
        n60 = control-ref of="Plot 4"() -> (w132:refnum<vi>)
        n61 = Bundle By Name(cluster=T4 {"Plot"=refnum, "Data"={"X"=[], "Predict"=[]}, "Indexe"={"X"=0, "Y"=1}, "Point Property"={"Style"=enum."Full circle", "Label Color"=[8978528, 4367871, 1985280]}} ("Parameters"), "Plot"=w104, "Data.X"=w30, "Data.Predict"=w107, "Indexe"=cluster{"X":i32, "Y":i32} {"X"=0, "Y"=1}, "Point Property"=cluster{"Style":T3, "Label Color":u32[]} {"Style"=enum."Full circle", "Label Color"=[3381759, 15694592]}) -> (w105:T4)
        n62 = call "2DPredictedClassification.vi"("error in"=w116, "Parameters"=w65) -> ("error out"=w89:errorcluster)  [unwired: 9 in]
        n63 = Bundle By Name(cluster=T4 {"Plot"=refnum, "Data"={"X"=[], "Predict"=[]}, "Indexe"={"X"=0, "Y"=1}, "Point Property"={"Style"=enum."Full circle", "Label Color"=[8978528, 4367871, 1985280]}} ("Parameters"), "Plot"=w132, "Data.X"=w30, "Data.Predict"=w134, "Indexe"=cluster{"X":i32, "Y":i32} {"X"=0, "Y"=1}, "Point Property"=cluster{"Style":T3, "Label Color":u32[]} {"Style"=enum."Full circle", "Label Color"=[3381759, 15694592]}) -> (w131:T4)
        n64 = call "2DPredictedClassification.vi"("error in"=w89, "Parameters"=w87) -> ("error out"=w106:errorcluster)  [unwired: 9 in]
        n65 = call "2DPredictedClassification.vi"("error in"=w106, "Parameters"=w105) -> ("error out"=w133:errorcluster)  [unwired: 9 in]
        n66 = call "2DPredictedClassification.vi"("error in"=w133, "Parameters"=w131) -> ("error out"=w32:errorcluster)  [unwired: 9 in]
      }
      frame 2 {
        # "Generate moons datasets and normalize dataset for easier parameter selection."
        n67 = Bundle By Name(cluster=T7 {"n_samples"="100", "shuffle"=TRUE, "noise"=-1.0, "random_state"=-1, "Returns"="X"} ("make_moons"), "n_samples"="1500", "noise"=0.05) -> (w144:T7)
        n68 = call "Moons.vi"("error in (no error)"=w137, "make_moons"=w144) -> ("error out"=w154:errorcluster, "Data"=w145:T9)  [unwired: 8 in]
        n69 = Unbundle By Name(w145) -> ("2DArray"=w155:string[][])
        n70 = call-poly "Processing Data.vi"("error in (no error)"=w154) -> ("error out"=w152:errorcluster, "StandardScaler.lvclass"=w153:refnum<class "StandardScaler.lvclass">)  [unwired: 9 in]
        n71 = call-dynamic "Fit Transform.vi"("Type X"=T1."Numeric Array", "error in (no error)"=w152, "X"=w155, "StandardScaler.lvclass"=w153) -> ("error out"=w150:errorcluster, "Data"=w149:T9, "StandardScaler.lvclass"=w151:refnum<class "StandardScaler.lvclass">)  [unwired: 5 in]
        n72 = Unbundle By Name(w149) -> ("2DArray"=w147:string[][])
        n73 = call-dynamic "ClosePython.vi"("error in (no error)"=w150, "Scikit-learn en entrée"=w151) -> ("error out"=w146:errorcluster)  [unwired: 8 in, 1 out]
        n74 = call "ArrayCharToString.vi"("TAB"=w147) -> ("Instruction"=w148:string)  [unwired: 10 in]
        n75 = call "StringToArrayFloat.vi"("entrée d'erreur (pas d'erreur)"=w146, "Return value"=w148) -> ("error IO"=w139:errorcluster, "2DArray"=w136:dbl[][])  [unwired: 7 in, 1 out]
        "noisy_moons" <- w136
      }
      frame 3 {
        # "Realize different linkage methods for hierarchical clustering on moons datasets."
        n76 = call-poly "Unsupervised.vi"("error in"=w157) -> ("error out"=w253:errorcluster, "out"=w254:refnum<class "AgglomerativeClustering.lvclass">)  [unwired: 9 in]
        n77 = Bundle By Name(cluster=T5 {"n_clusters"={"n_clusters_type"="int", "n_clusters_int"=0.0}, "affinity"={"affinity_type"="euclidean", "affinity_function"="metric_function"}, "memory"="", "connectivity"={"connectivity_type"="None", "connectivity_list"=[]}, "compute_full_tree"={"compute_full_tree_type"="auto", "compute_full_tree_bool"=FALSE}, "linkage"="ward", "distance_threshold"={"distance_threshold_type"="None", "distance_threshold_float"=0.0}, "compute_distances"=FALSE} ("output cluster"), "n_clusters"=T6 {"n_clusters_type"="int", "n_clusters_int"=2.0}, "linkage"="ward") -> (w230:T5)
        n78 = Bundle By Name(cluster=w230, "linkage"="complete") -> (w215:T5)
        n79 = call-dynamic "init.vi"("error in (no error)"=w253, "Model en entrée"=w254) -> ("error out"=w252:errorcluster, "Model en sortie"=w258:refnum<class "AgglomerativeClustering.lvclass">)  [unwired: 8 in]
        n80 = Bundle By Name(cluster=w215, "linkage"="average") -> (w197:T5)
        n81 = Bundle By Name(cluster=w197, "linkage"="single") -> (w199:T5)
        n82 = property class="AgglomerativeClustering.lvclass"(reference=w258, error in=w252, "accessors:R/W params"=w230) -> (reference out=w257:refnum<class "AgglomerativeClustering.lvclass">, error out=w251:errorcluster)
        n83 = call-dynamic "set_params.vi"("error in (no error)"=w251, "AgglomerativeClustering.lvclass 2"=w257) -> ("error out"=w250:errorcluster, "AgglomerativeClustering.lvclass"=w256:refnum<class "AgglomerativeClustering.lvclass">)  [unwired: 8 in]
        n84 = property class="AgglomerativeClustering.lvclass"(reference=w256, error in=w250, "accessors:R/W X"=w156) -> (reference out=w259:refnum<class "AgglomerativeClustering.lvclass">, error out=w249:errorcluster)
        n85 = call-dynamic "fit.vi"("error in (no error)"=w249, "AgglomerativeClustering.lvclass 2"=w259) -> ("error out"=w248:errorcluster, "AgglomerativeClustering.lvclass"=w255:refnum<class "AgglomerativeClustering.lvclass">)  [unwired: 8 in]
        n86 = call-dynamic "get_attributes.vi"("error in (no error)"=w248, "AgglomerativeClustering.lvclass 2"=w255) -> ("error out"=w243:errorcluster, "AgglomerativeClustering.lvclass"=w244:refnum<class "AgglomerativeClustering.lvclass">)  [unwired: 8 in]
        n87 = property class="AgglomerativeClustering.lvclass"(reference=w244, error in=w243) -> (reference out=w229:refnum<class "AgglomerativeClustering.lvclass">, error out=w228:errorcluster, "accessors:R/W attributes"=w247:T10)
        n88 = property class="AgglomerativeClustering.lvclass"(reference=w229, error in=w228, "accessors:R/W params"=w215) -> (reference out=w232:refnum<class "AgglomerativeClustering.lvclass">, error out=w235:errorcluster)
        n89 = call-dynamic "set_params.vi"("error in (no error)"=w235, "AgglomerativeClustering.lvclass 2"=w232) -> ("error out"=w236:errorcluster, "AgglomerativeClustering.lvclass"=w233:refnum<class "AgglomerativeClustering.lvclass">)  [unwired: 8 in]
        n90 = property class="AgglomerativeClustering.lvclass"(reference=w233, error in=w236, "accessors:R/W X"=w156) -> (reference out=w231:refnum<class "AgglomerativeClustering.lvclass">, error out=w237:errorcluster)
        n91 = call-dynamic "fit.vi"("error in (no error)"=w237, "AgglomerativeClustering.lvclass 2"=w231) -> ("error out"=w238:errorcluster, "AgglomerativeClustering.lvclass"=w234:refnum<class "AgglomerativeClustering.lvclass">)  [unwired: 8 in]
        n92 = call-dynamic "get_attributes.vi"("error in (no error)"=w238, "AgglomerativeClustering.lvclass 2"=w234) -> ("error out"=w240:errorcluster, "AgglomerativeClustering.lvclass"=w239:refnum<class "AgglomerativeClustering.lvclass">)  [unwired: 8 in]
        n93 = property class="AgglomerativeClustering.lvclass"(reference=w239, error in=w240) -> (reference out=w214:refnum<class "AgglomerativeClustering.lvclass">, error out=w213:errorcluster, "accessors:R/W attributes"=w225:T10)
        n94 = property class="AgglomerativeClustering.lvclass"(reference=w214, error in=w213, "accessors:R/W params"=w197) -> (reference out=w212:refnum<class "AgglomerativeClustering.lvclass">, error out=w220:errorcluster)
        n95 = call-dynamic "set_params.vi"("error in (no error)"=w220, "AgglomerativeClustering.lvclass 2"=w212) -> ("error out"=w219:errorcluster, "AgglomerativeClustering.lvclass"=w211:refnum<class "AgglomerativeClustering.lvclass">)  [unwired: 8 in]
        n96 = property class="AgglomerativeClustering.lvclass"(reference=w211, error in=w219, "accessors:R/W X"=w156) -> (reference out=w194:refnum<class "AgglomerativeClustering.lvclass">, error out=w218:errorcluster)
        n97 = call-dynamic "fit.vi"("error in (no error)"=w218, "AgglomerativeClustering.lvclass 2"=w194) -> ("error out"=w217:errorcluster, "AgglomerativeClustering.lvclass"=w193:refnum<class "AgglomerativeClustering.lvclass">)  [unwired: 8 in]
        n98 = call-dynamic "get_attributes.vi"("error in (no error)"=w217, "AgglomerativeClustering.lvclass 2"=w193) -> ("error out"=w216:errorcluster, "AgglomerativeClustering.lvclass"=w192:refnum<class "AgglomerativeClustering.lvclass">)  [unwired: 8 in]
        n99 = property class="AgglomerativeClustering.lvclass"(reference=w192, error in=w216) -> (reference out=w191:refnum<class "AgglomerativeClustering.lvclass">, error out=w190:errorcluster, "accessors:R/W attributes"=w210:T10)
        n100 = property class="AgglomerativeClustering.lvclass"(reference=w191, error in=w190, "accessors:R/W params"=w199) -> (reference out=w196:refnum<class "AgglomerativeClustering.lvclass">, error out=w200:errorcluster)
        n101 = call-dynamic "set_params.vi"("error in (no error)"=w200, "AgglomerativeClustering.lvclass 2"=w196) -> ("error out"=w184:errorcluster, "AgglomerativeClustering.lvclass"=w185:refnum<class "AgglomerativeClustering.lvclass">)  [unwired: 8 in]
        n102 = property class="AgglomerativeClustering.lvclass"(reference=w185, error in=w184, "accessors:R/W X"=w156) -> (reference out=w186:refnum<class "AgglomerativeClustering.lvclass">, error out=w201:errorcluster)
        n103 = call-dynamic "fit.vi"("error in (no error)"=w201, "AgglomerativeClustering.lvclass 2"=w186) -> ("error out"=w202:errorcluster, "AgglomerativeClustering.lvclass"=w187:refnum<class "AgglomerativeClustering.lvclass">)  [unwired: 8 in]
        n104 = call-dynamic "get_attributes.vi"("error in (no error)"=w202, "AgglomerativeClustering.lvclass 2"=w187) -> ("error out"=w203:errorcluster, "AgglomerativeClustering.lvclass"=w188:refnum<class "AgglomerativeClustering.lvclass">)  [unwired: 8 in]
        n105 = property class="AgglomerativeClustering.lvclass"(reference=w188, error in=w203) -> (reference out=w189:refnum<class "AgglomerativeClustering.lvclass">, error out=w198:errorcluster, "accessors:R/W attributes"=w181:T10)
        n106 = call-dynamic "closeSession.vi"("error in"=w198, "Python en entrée"=w189) -> ("error out"=w195:errorcluster)  [unwired: 8 in, 1 out]
        n107 = Unbundle By Name(w247) -> ("labels_"=w260:dbl[])
        n108 = Unbundle By Name(w225) -> ("labels_"=w226:dbl[])
        n109 = Unbundle By Name(w210) -> ("labels_"=w208:dbl[])
        n110 = Unbundle By Name(w181) -> ("labels_"=w183:dbl[])
        n111 = Build Array(w260) -> (w242:dbl[][])
        n112 = Build Array(w226) -> (w227:dbl[][])
        n113 = Build Array(w208) -> (w209:dbl[][])
        n114 = Build Array(w183) -> (w182:dbl[][])
        n115 = Transpose 2D Array(2D array=w242) -> (transposed array=w241:dbl[][])
        n116 = Transpose 2D Array(2D array=w227) -> (transposed array=w221:dbl[][])
        n117 = Transpose 2D Array(2D array=w209) -> (transposed array=w204:dbl[][])
        n118 = Transpose 2D Array(2D array=w182) -> (transposed array=w177:dbl[][])
        n119 = control-ref of="Plot 8"() -> (w246:refnum<vi>)
        n120 = control-ref of="Plot 7"() -> (w223:refnum<vi>)
        n121 = Bundle By Name(cluster=T4 {"Plot"=refnum, "Data"={"X"=[], "Predict"=[]}, "Indexe"={"X"=0, "Y"=1}, "Point Property"={"Style"=enum."Full circle", "Label Color"=[8978528, 4367871, 1985280]}} ("Parameters"), "Plot"=w246, "Data.X"=w156, "Data.Predict"=w241, "Indexe"=cluster{"X":i32, "Y":i32} {"X"=0, "Y"=1}, "Point Property"=cluster{"Style":T3, "Label Color":u32[]} {"Style"=enum."Full circle", "Label Color"=[3381759, 15694592]}) -> (w245:T4)
        n122 = control-ref of="Plot 6"() -> (w207:refnum<vi>)
        n123 = Bundle By Name(cluster=T4 {"Plot"=refnum, "Data"={"X"=[], "Predict"=[]}, "Indexe"={"X"=0, "Y"=1}, "Point Property"={"Style"=enum."Full circle", "Label Color"=[8978528, 4367871, 1985280]}} ("Parameters"), "Plot"=w223, "Data.X"=w156, "Data.Predict"=w221, "Indexe"=cluster{"X":i32, "Y":i32} {"X"=0, "Y"=1}, "Point Property"=cluster{"Style":T3, "Label Color":u32[]} {"Style"=enum."Full circle", "Label Color"=[3381759, 15694592]}) -> (w224:T4)
        n124 = control-ref of="Plot 5"() -> (w179:refnum<vi>)
        n125 = call "2DPredictedClassification.vi"("error in"=w195, "Parameters"=w245) -> ("error out"=w222:errorcluster)  [unwired: 9 in]
        n126 = Bundle By Name(cluster=T4 {"Plot"=refnum, "Data"={"X"=[], "Predict"=[]}, "Indexe"={"X"=0, "Y"=1}, "Point Property"={"Style"=enum."Full circle", "Label Color"=[8978528, 4367871, 1985280]}} ("Parameters"), "Plot"=w207, "Data.X"=w156, "Data.Predict"=w204, "Indexe"=cluster{"X":i32, "Y":i32} {"X"=0, "Y"=1}, "Point Property"=cluster{"Style":T3, "Label Color":u32[]} {"Style"=enum."Full circle", "Label Color"=[3381759, 15694592]}) -> (w206:T4)
        n127 = Bundle By Name(cluster=T4 {"Plot"=refnum, "Data"={"X"=[], "Predict"=[]}, "Indexe"={"X"=0, "Y"=1}, "Point Property"={"Style"=enum."Full circle", "Label Color"=[8978528, 4367871, 1985280]}} ("Parameters"), "Plot"=w179, "Data.X"=w156, "Data.Predict"=w177, "Indexe"=cluster{"X":i32, "Y":i32} {"X"=0, "Y"=1}, "Point Property"=cluster{"Style":T3, "Label Color":u32[]} {"Style"=enum."Full circle", "Label Color"=[3381759, 15694592]}) -> (w180:T4)
        n128 = call "2DPredictedClassification.vi"("error in"=w222, "Parameters"=w224) -> ("error out"=w205:errorcluster)  [unwired: 9 in]
        n129 = call "2DPredictedClassification.vi"("error in"=w205, "Parameters"=w206) -> ("error out"=w178:errorcluster)  [unwired: 9 in]
        n130 = call "2DPredictedClassification.vi"("error in"=w178, "Parameters"=w180) -> ("error out"=w162:errorcluster)  [unwired: 9 in]
      }
      frame 4 {
        # "Generate blobs datasets and normalize dataset for easier parameter selection."
        n131 = Bundle By Name(cluster=T8 {"n_samples"=[100], "n_features"=2, "centers"=[], "cluster_std"=[1.0], "centermin"=-10.0, "centermax"=10.0, "shuffle"=TRUE, "random_state"=-1, "Returns"="X"} ("make_blobs"), "n_samples"=i32[] [1500], "random_state"=8) -> (w270:T8)
        n132 = call "Blobs.vi"("error in (no error)"=w263, "make_blobs"=w270) -> ("error out"=w281:errorcluster, "Data"=w271:T9)  [unwired: 8 in]
        n133 = Unbundle By Name(w271) -> ("2DArray"=w280:string[][])
        n134 = call-poly "Processing Data.vi"("error in (no error)"=w281) -> ("error out"=w273:errorcluster, "StandardScaler.lvclass"=w272:refnum<class "StandardScaler.lvclass">)  [unwired: 9 in]
        n135 = call-dynamic "Fit Transform.vi"("Type X"=T1."Numeric Array", "error in (no error)"=w273, "X"=w280, "StandardScaler.lvclass"=w272) -> ("error out"=w275:errorcluster, "Data"=w276:T9, "StandardScaler.lvclass"=w274:refnum<class "StandardScaler.lvclass">)  [unwired: 5 in]
        n136 = Unbundle By Name(w276) -> ("2DArray"=w278:string[][])
        n137 = call-dynamic "ClosePython.vi"("error in (no error)"=w275, "Scikit-learn en entrée"=w274) -> ("error out"=w279:errorcluster)  [unwired: 8 in, 1 out]
        n138 = call "ArrayCharToString.vi"("TAB"=w278) -> ("Instruction"=w277:string)  [unwired: 10 in]
        n139 = call "StringToArrayFloat.vi"("entrée d'erreur (pas d'erreur)"=w279, "Return value"=w277) -> ("error IO"=w265:errorcluster, "2DArray"=w262:dbl[][])  [unwired: 7 in, 1 out]
        "blobs" <- w262
      }
      frame 5 {
        # "Realize different linkage methods for hierarchical clustering on blobs datasets."
        n140 = call-poly "Unsupervised.vi"("error in"=w283) -> ("error out"=w310:errorcluster, "out"=w309:refnum<class "AgglomerativeClustering.lvclass">)  [unwired: 9 in]
        n141 = Bundle By Name(cluster=T5 {"n_clusters"={"n_clusters_type"="int", "n_clusters_int"=0.0}, "affinity"={"affinity_type"="euclidean", "affinity_function"="metric_function"}, "memory"="", "connectivity"={"connectivity_type"="None", "connectivity_list"=[]}, "compute_full_tree"={"compute_full_tree_type"="auto", "compute_full_tree_bool"=FALSE}, "linkage"="ward", "distance_threshold"={"distance_threshold_type"="None", "distance_threshold_float"=0.0}, "compute_distances"=FALSE} ("output cluster"), "n_clusters"=T6 {"n_clusters_type"="int", "n_clusters_int"=3.0}, "linkage"="ward") -> (w333:T5)
        n142 = Bundle By Name(cluster=w333, "linkage"="complete") -> (w348:T5)
        n143 = call-dynamic "init.vi"("error in (no error)"=w310, "Model en entrée"=w309) -> ("error out"=w311:errorcluster, "Model en sortie"=w305:refnum<class "AgglomerativeClustering.lvclass">)  [unwired: 8 in]
        n144 = Bundle By Name(cluster=w348, "linkage"="average") -> (w366:T5)
        n145 = Bundle By Name(cluster=w366, "linkage"="single") -> (w364:T5)
        n146 = property class="AgglomerativeClustering.lvclass"(reference=w305, error in=w311, "accessors:R/W params"=w333) -> (reference out=w306:refnum<class "AgglomerativeClustering.lvclass">, error out=w312:errorcluster)
        n147 = call-dynamic "set_params.vi"("error in (no error)"=w312, "AgglomerativeClustering.lvclass 2"=w306) -> ("error out"=w313:errorcluster, "AgglomerativeClustering.lvclass"=w307:refnum<class "AgglomerativeClustering.lvclass">)  [unwired: 8 in]
        n148 = property class="AgglomerativeClustering.lvclass"(reference=w307, error in=w313, "accessors:R/W X"=w282) -> (reference out=w304:refnum<class "AgglomerativeClustering.lvclass">, error out=w314:errorcluster)
        n149 = call-dynamic "fit.vi"("error in (no error)"=w314, "AgglomerativeClustering.lvclass 2"=w304) -> ("error out"=w315:errorcluster, "AgglomerativeClustering.lvclass"=w308:refnum<class "AgglomerativeClustering.lvclass">)  [unwired: 8 in]
        n150 = call-dynamic "get_attributes.vi"("error in (no error)"=w315, "AgglomerativeClustering.lvclass 2"=w308) -> ("error out"=w320:errorcluster, "AgglomerativeClustering.lvclass"=w319:refnum<class "AgglomerativeClustering.lvclass">)  [unwired: 8 in]
        n151 = property class="AgglomerativeClustering.lvclass"(reference=w319, error in=w320) -> (reference out=w334:refnum<class "AgglomerativeClustering.lvclass">, error out=w335:errorcluster, "accessors:R/W attributes"=w316:T10)
        n152 = property class="AgglomerativeClustering.lvclass"(reference=w334, error in=w335, "accessors:R/W params"=w348) -> (reference out=w331:refnum<class "AgglomerativeClustering.lvclass">, error out=w328:errorcluster)
        n153 = call-dynamic "set_params.vi"("error in (no error)"=w328, "AgglomerativeClustering.lvclass 2"=w331) -> ("error out"=w327:errorcluster, "AgglomerativeClustering.lvclass"=w330:refnum<class "AgglomerativeClustering.lvclass">)  [unwired: 8 in]
        n154 = property class="AgglomerativeClustering.lvclass"(reference=w330, error in=w327, "accessors:R/W X"=w282) -> (reference out=w332:refnum<class "AgglomerativeClustering.lvclass">, error out=w326:errorcluster)
        n155 = call-dynamic "fit.vi"("error in (no error)"=w326, "AgglomerativeClustering.lvclass 2"=w332) -> ("error out"=w325:errorcluster, "AgglomerativeClustering.lvclass"=w329:refnum<class "AgglomerativeClustering.lvclass">)  [unwired: 8 in]
        n156 = call-dynamic "get_attributes.vi"("error in (no error)"=w325, "AgglomerativeClustering.lvclass 2"=w329) -> ("error out"=w323:errorcluster, "AgglomerativeClustering.lvclass"=w324:refnum<class "AgglomerativeClustering.lvclass">)  [unwired: 8 in]
        n157 = property class="AgglomerativeClustering.lvclass"(reference=w324, error in=w323) -> (reference out=w349:refnum<class "AgglomerativeClustering.lvclass">, error out=w350:errorcluster, "accessors:R/W attributes"=w338:T10)
        n158 = property class="AgglomerativeClustering.lvclass"(reference=w349, error in=w350, "accessors:R/W params"=w366) -> (reference out=w351:refnum<class "AgglomerativeClustering.lvclass">, error out=w343:errorcluster)
        n159 = call-dynamic "set_params.vi"("error in (no error)"=w343, "AgglomerativeClustering.lvclass 2"=w351) -> ("error out"=w344:errorcluster, "AgglomerativeClustering.lvclass"=w352:refnum<class "AgglomerativeClustering.lvclass">)  [unwired: 8 in]
        n160 = property class="AgglomerativeClustering.lvclass"(reference=w352, error in=w344, "accessors:R/W X"=w282) -> (reference out=w369:refnum<class "AgglomerativeClustering.lvclass">, error out=w345:errorcluster)
        n161 = call-dynamic "fit.vi"("error in (no error)"=w345, "AgglomerativeClustering.lvclass 2"=w369) -> ("error out"=w346:errorcluster, "AgglomerativeClustering.lvclass"=w370:refnum<class "AgglomerativeClustering.lvclass">)  [unwired: 8 in]
        n162 = call-dynamic "get_attributes.vi"("error in (no error)"=w346, "AgglomerativeClustering.lvclass 2"=w370) -> ("error out"=w347:errorcluster, "AgglomerativeClustering.lvclass"=w371:refnum<class "AgglomerativeClustering.lvclass">)  [unwired: 8 in]
        n163 = property class="AgglomerativeClustering.lvclass"(reference=w371, error in=w347) -> (reference out=w372:refnum<class "AgglomerativeClustering.lvclass">, error out=w373:errorcluster, "accessors:R/W attributes"=w353:T10)
        n164 = property class="AgglomerativeClustering.lvclass"(reference=w372, error in=w373, "accessors:R/W params"=w364) -> (reference out=w367:refnum<class "AgglomerativeClustering.lvclass">, error out=w363:errorcluster)
        n165 = call-dynamic "set_params.vi"("error in (no error)"=w363, "AgglomerativeClustering.lvclass 2"=w367) -> ("error out"=w379:errorcluster, "AgglomerativeClustering.lvclass"=w378:refnum<class "AgglomerativeClustering.lvclass">)  [unwired: 8 in]
        n166 = property class="AgglomerativeClustering.lvclass"(reference=w378, error in=w379, "accessors:R/W X"=w282) -> (reference out=w377:refnum<class "AgglomerativeClustering.lvclass">, error out=w362:errorcluster)
        n167 = call-dynamic "fit.vi"("error in (no error)"=w362, "AgglomerativeClustering.lvclass 2"=w377) -> ("error out"=w361:errorcluster, "AgglomerativeClustering.lvclass"=w376:refnum<class "AgglomerativeClustering.lvclass">)  [unwired: 8 in]
        n168 = call-dynamic "get_attributes.vi"("error in (no error)"=w361, "AgglomerativeClustering.lvclass 2"=w376) -> ("error out"=w360:errorcluster, "AgglomerativeClustering.lvclass"=w375:refnum<class "AgglomerativeClustering.lvclass">)  [unwired: 8 in]
        n169 = property class="AgglomerativeClustering.lvclass"(reference=w375, error in=w360) -> (reference out=w374:refnum<class "AgglomerativeClustering.lvclass">, error out=w365:errorcluster, "accessors:R/W attributes"=w382:T10)
        n170 = call-dynamic "closeSession.vi"("error in"=w365, "Python en entrée"=w374) -> ("error out"=w368:errorcluster)  [unwired: 8 in, 1 out]
        n171 = Unbundle By Name(w353) -> ("labels_"=w355:dbl[])
        n172 = Unbundle By Name(w316) -> ("labels_"=w303:dbl[])
        n173 = Unbundle By Name(w338) -> ("labels_"=w337:dbl[])
        n174 = Unbundle By Name(w382) -> ("labels_"=w380:dbl[])
        n175 = Build Array(w303) -> (w321:dbl[][])
        n176 = Build Array(w355) -> (w354:dbl[][])
        n177 = Build Array(w337) -> (w336:dbl[][])
        n178 = Build Array(w380) -> (w381:dbl[][])
        n179 = Transpose 2D Array(2D array=w354) -> (transposed array=w359:dbl[][])
        n180 = Transpose 2D Array(2D array=w321) -> (transposed array=w322:dbl[][])
        n181 = Transpose 2D Array(2D array=w336) -> (transposed array=w342:dbl[][])
        n182 = Transpose 2D Array(2D array=w381) -> (transposed array=w386:dbl[][])
        n183 = control-ref of="Plot 12"() -> (w317:refnum<vi>)
        n184 = Bundle By Name(cluster=T4 {"Plot"=refnum, "Data"={"X"=[], "Predict"=[]}, "Indexe"={"X"=0, "Y"=1}, "Point Property"={"Style"=enum."Full circle", "Label Color"=[8978528, 4367871, 1985280]}} ("Parameters"), "Plot"=w317, "Data.X"=w282, "Data.Predict"=w322, "Indexe"=cluster{"X":i32, "Y":i32} {"X"=0, "Y"=1}, "Point Property"=cluster{"Style":T3, "Label Color":u32[]} {"Style"=enum."Full circle", "Label Color"=[3381759, 15694592, 51218]}) -> (w318:T4)
        n185 = control-ref of="Plot 11"() -> (w340:refnum<vi>)
        n186 = control-ref of="Plot 10"() -> (w356:refnum<vi>)
        n187 = Bundle By Name(cluster=T4 {"Plot"=refnum, "Data"={"X"=[], "Predict"=[]}, "Indexe"={"X"=0, "Y"=1}, "Point Property"={"Style"=enum."Full circle", "Label Color"=[8978528, 4367871, 1985280]}} ("Parameters"), "Plot"=w340, "Data.X"=w282, "Data.Predict"=w342, "Indexe"=cluster{"X":i32, "Y":i32} {"X"=0, "Y"=1}, "Point Property"=cluster{"Style":T3, "Label Color":u32[]} {"Style"=enum."Full circle", "Label Color"=[3381759, 15694592, 51218]}) -> (w339:T4)
        n188 = control-ref of="Plot 9"() -> (w384:refnum<vi>)
        n189 = call "2DPredictedClassification.vi"("error in"=w368, "Parameters"=w318) -> ("error out"=w341:errorcluster)  [unwired: 9 in]
        n190 = Bundle By Name(cluster=T4 {"Plot"=refnum, "Data"={"X"=[], "Predict"=[]}, "Indexe"={"X"=0, "Y"=1}, "Point Property"={"Style"=enum."Full circle", "Label Color"=[8978528, 4367871, 1985280]}} ("Parameters"), "Plot"=w356, "Data.X"=w282, "Data.Predict"=w359, "Indexe"=cluster{"X":i32, "Y":i32} {"X"=0, "Y"=1}, "Point Property"=cluster{"Style":T3, "Label Color":u32[]} {"Style"=enum."Full circle", "Label Color"=[3381759, 15694592, 51218]}) -> (w357:T4)
        n191 = Bundle By Name(cluster=T4 {"Plot"=refnum, "Data"={"X"=[], "Predict"=[]}, "Indexe"={"X"=0, "Y"=1}, "Point Property"={"Style"=enum."Full circle", "Label Color"=[8978528, 4367871, 1985280]}} ("Parameters"), "Plot"=w384, "Data.X"=w282, "Data.Predict"=w386, "Indexe"=cluster{"X":i32, "Y":i32} {"X"=0, "Y"=1}, "Point Property"=cluster{"Style":T3, "Label Color":u32[]} {"Style"=enum."Full circle", "Label Color"=[3381759, 15694592, 51218]}) -> (w383:T4)
        n192 = call "2DPredictedClassification.vi"("error in"=w341, "Parameters"=w339) -> ("error out"=w358:errorcluster)  [unwired: 9 in]
        n193 = call "2DPredictedClassification.vi"("error in"=w358, "Parameters"=w357) -> ("error out"=w385:errorcluster)  [unwired: 9 in]
        n194 = call "2DPredictedClassification.vi"("error in"=w385, "Parameters"=w383) -> ("error out"=w288:errorcluster)  [unwired: 9 in]
      }
      frame 6 {
        # "Generate anisotropicly datasets and normalize dataset for easier parameter selection."
        n195 = Bundle By Name(cluster=T8 {"n_samples"=[100], "n_features"=2, "centers"=[], "cluster_std"=[1.0], "centermin"=-10.0, "centermax"=10.0, "shuffle"=TRUE, "random_state"=-1, "Returns"="X"} ("make_blobs"), "n_samples"=i32[] [1500], "random_state"=170) -> (w410:T8)
        n196 = Bundle By Name(cluster=T8 {"n_samples"=[100], "n_features"=2, "centers"=[], "cluster_std"=[1.0], "centermin"=-10.0, "centermax"=10.0, "shuffle"=TRUE, "random_state"=-1, "Returns"="X"} ("make_blobs"), "n_samples"=i32[] [1500], "random_state"=170) -> (w405:T8)
        n197 = call "Blobs.vi"("error in (no error)"=w391, "make_blobs"=w410) -> ("error out"=w413:errorcluster, "Data"=w412:T9)  [unwired: 8 in]
        n198 = call "Blobs.vi"("error in (no error)"=w391, "make_blobs"=w405) -> ("error out"=w401:errorcluster, "Data"=w402:T9)  [unwired: 8 in]
        n199 = Unbundle By Name(w412) -> ("1DArray"=w414:string[])
        n200 = Unbundle By Name(w402) -> ("2DArray"=w403:string[][])
        n201 = Build Array(w414) -> (w415:string[][])
        n202 = call "ArrayCharToString.vi"("TAB"=w403) -> ("Instruction"=w404:string)  [unwired: 10 in]
        n203 = call "ArrayCharToString.vi"("TAB"=w415) -> ("Instruction"=w411:string)  [unwired: 10 in]
        n204 = call "StringToArrayFloat.vi"("entrée d'erreur (pas d'erreur)"=w413, "Return value"=w411) -> ("error IO"=w432:errorcluster, "1DArray"=w416:dbl[])  [unwired: 7 in, 1 out]
        n205 = call "StringToArrayFloat.vi"("entrée d'erreur (pas d'erreur)"=w401, "Return value"=w404) -> ("error IO"=w431:errorcluster, "2DArray"=w409:dbl[][])  [unwired: 7 in, 1 out]
        n206 = call-poly <vilib>:"Array To Matrix.vi"("Real 2D Array"=dbl[][] [[0.6, -0.6], [-0.4, 0.8]]) -> ("Real Matrix"=w407:T11)
        n207 = call-poly <vilib>:"Array To Matrix.vi"("Real 2D Array"=w409) -> ("Real Matrix"=w406:T11)
        n208 = call-poly <vilib>:"A x B.vi"("B"=w407, "A"=w406) -> ("A x B"=w408:T11)  [unwired: 1 out]
        n209 = call-poly <vilib>:"Matrix To Array.vi"("Real Matrix"=w408) -> ("Real 2D Array"=w417:dbl[][])
        "X_aniso" <- w417
        n210 = Array Size(array=w417) -> (size(s)=w418:i32[])
        n211 = Index Array(array=w418, index=1) -> (element=w419:i32)
        n212 = Insert Into Array(array=w417, index (col)=w419, new element=w416) -> (w428:dbl[][])  [unwired: 1 in]
        n213 = Merge Errors(w431, w432) -> (w430:errorcluster)
        n214 = call "ArrayFloatToString.vi"("2D Data"=w428) -> ("Array"=w429:string[][])  [unwired: 9 in, 1 out]
        n215 = call-poly "Processing Data.vi"("error in (no error)"=w430) -> ("error out"=w426:errorcluster, "StandardScaler.lvclass"=w427:refnum<class "StandardScaler.lvclass">)  [unwired: 9 in]
        n216 = call-dynamic "Fit Transform.vi"("Type X"=T1."Numeric Array", "error in (no error)"=w426, "X"=w429, "StandardScaler.lvclass"=w427) -> ("error out"=w424:errorcluster, "Data"=w423:T9, "StandardScaler.lvclass"=w425:refnum<class "StandardScaler.lvclass">)  [unwired: 5 in]
        n217 = Unbundle By Name(w423) -> ("2DArray"=w421:string[][])
        n218 = call-dynamic "ClosePython.vi"("error in (no error)"=w424, "Scikit-learn en entrée"=w425) -> ("error out"=w420:errorcluster)  [unwired: 8 in, 1 out]
        n219 = call "ArrayCharToString.vi"("TAB"=w421) -> ("Instruction"=w422:string)  [unwired: 10 in]
        n220 = call "StringToArrayFloat.vi"("entrée d'erreur (pas d'erreur)"=w420, "Return value"=w422) -> ("error IO"=w390:errorcluster, "2DArray"=w388:dbl[][])  [unwired: 7 in, 1 out]
        "aniso" <- w388
      }
      frame 7 {
        # "Realize different linkage methods for hierarchical clustering on anisotropicly datasets."
        n221 = call-poly "Unsupervised.vi"("error in"=w434) -> ("error out"=w530:errorcluster, "out"=w531:refnum<class "AgglomerativeClustering.lvclass">)  [unwired: 9 in]
        n222 = Bundle By Name(cluster=T5 {"n_clusters"={"n_clusters_type"="int", "n_clusters_int"=0.0}, "affinity"={"affinity_type"="euclidean", "affinity_function"="metric_function"}, "memory"="", "connectivity"={"connectivity_type"="None", "connectivity_list"=[]}, "compute_full_tree"={"compute_full_tree_type"="auto", "compute_full_tree_bool"=FALSE}, "linkage"="ward", "distance_threshold"={"distance_threshold_type"="None", "distance_threshold_float"=0.0}, "compute_distances"=FALSE} ("output cluster"), "n_clusters"=T6 {"n_clusters_type"="int", "n_clusters_int"=3.0}, "linkage"="ward") -> (w507:T5)
        n223 = call-dynamic "init.vi"("error in (no error)"=w530, "Model en entrée"=w531) -> ("error out"=w529:errorcluster, "Model en sortie"=w535:refnum<class "AgglomerativeClustering.lvclass">)  [unwired: 8 in]
        n224 = Bundle By Name(cluster=w507, "linkage"="complete") -> (w492:T5)
        n225 = Bundle By Name(cluster=w492, "linkage"="average") -> (w474:T5)
        n226 = Bundle By Name(cluster=w474, "linkage"="single") -> (w476:T5)
        n227 = property class="AgglomerativeClustering.lvclass"(reference=w535, error in=w529, "accessors:R/W params"=w507) -> (reference out=w534:refnum<class "AgglomerativeClustering.lvclass">, error out=w528:errorcluster)
        n228 = call-dynamic "set_params.vi"("error in (no error)"=w528, "AgglomerativeClustering.lvclass 2"=w534) -> ("error out"=w527:errorcluster, "AgglomerativeClustering.lvclass"=w533:refnum<class "AgglomerativeClustering.lvclass">)  [unwired: 8 in]
        n229 = property class="AgglomerativeClustering.lvclass"(reference=w533, error in=w527, "accessors:R/W X"=w433) -> (reference out=w536:refnum<class "AgglomerativeClustering.lvclass">, error out=w526:errorcluster)
        n230 = call-dynamic "fit.vi"("error in (no error)"=w526, "AgglomerativeClustering.lvclass 2"=w536) -> ("error out"=w525:errorcluster, "AgglomerativeClustering.lvclass"=w532:refnum<class "AgglomerativeClustering.lvclass">)  [unwired: 8 in]
        n231 = call-dynamic "get_attributes.vi"("error in (no error)"=w525, "AgglomerativeClustering.lvclass 2"=w532) -> ("error out"=w520:errorcluster, "AgglomerativeClustering.lvclass"=w521:refnum<class "AgglomerativeClustering.lvclass">)  [unwired: 8 in]
        n232 = property class="AgglomerativeClustering.lvclass"(reference=w521, error in=w520) -> (reference out=w506:refnum<class "AgglomerativeClustering.lvclass">, error out=w505:errorcluster, "accessors:R/W attributes"=w524:T10)
        n233 = property class="AgglomerativeClustering.lvclass"(reference=w506, error in=w505, "accessors:R/W params"=w492) -> (reference out=w509:refnum<class "AgglomerativeClustering.lvclass">, error out=w512:errorcluster)
        n234 = call-dynamic "set_params.vi"("error in (no error)"=w512, "AgglomerativeClustering.lvclass 2"=w509) -> ("error out"=w513:errorcluster, "AgglomerativeClustering.lvclass"=w510:refnum<class "AgglomerativeClustering.lvclass">)  [unwired: 8 in]
        n235 = property class="AgglomerativeClustering.lvclass"(reference=w510, error in=w513, "accessors:R/W X"=w433) -> (reference out=w508:refnum<class "AgglomerativeClustering.lvclass">, error out=w514:errorcluster)
        n236 = call-dynamic "fit.vi"("error in (no error)"=w514, "AgglomerativeClustering.lvclass 2"=w508) -> ("error out"=w515:errorcluster, "AgglomerativeClustering.lvclass"=w511:refnum<class "AgglomerativeClustering.lvclass">)  [unwired: 8 in]
        n237 = call-dynamic "get_attributes.vi"("error in (no error)"=w515, "AgglomerativeClustering.lvclass 2"=w511) -> ("error out"=w517:errorcluster, "AgglomerativeClustering.lvclass"=w516:refnum<class "AgglomerativeClustering.lvclass">)  [unwired: 8 in]
        n238 = property class="AgglomerativeClustering.lvclass"(reference=w516, error in=w517) -> (reference out=w491:refnum<class "AgglomerativeClustering.lvclass">, error out=w490:errorcluster, "accessors:R/W attributes"=w502:T10)
        n239 = property class="AgglomerativeClustering.lvclass"(reference=w491, error in=w490, "accessors:R/W params"=w474) -> (reference out=w489:refnum<class "AgglomerativeClustering.lvclass">, error out=w497:errorcluster)
        n240 = call-dynamic "set_params.vi"("error in (no error)"=w497, "AgglomerativeClustering.lvclass 2"=w489) -> ("error out"=w496:errorcluster, "AgglomerativeClustering.lvclass"=w488:refnum<class "AgglomerativeClustering.lvclass">)  [unwired: 8 in]
        n241 = property class="AgglomerativeClustering.lvclass"(reference=w488, error in=w496, "accessors:R/W X"=w433) -> (reference out=w471:refnum<class "AgglomerativeClustering.lvclass">, error out=w495:errorcluster)
        n242 = call-dynamic "fit.vi"("error in (no error)"=w495, "AgglomerativeClustering.lvclass 2"=w471) -> ("error out"=w494:errorcluster, "AgglomerativeClustering.lvclass"=w470:refnum<class "AgglomerativeClustering.lvclass">)  [unwired: 8 in]
        n243 = call-dynamic "get_attributes.vi"("error in (no error)"=w494, "AgglomerativeClustering.lvclass 2"=w470) -> ("error out"=w493:errorcluster, "AgglomerativeClustering.lvclass"=w469:refnum<class "AgglomerativeClustering.lvclass">)  [unwired: 8 in]
        n244 = property class="AgglomerativeClustering.lvclass"(reference=w469, error in=w493) -> (reference out=w468:refnum<class "AgglomerativeClustering.lvclass">, error out=w467:errorcluster, "accessors:R/W attributes"=w487:T10)
        n245 = property class="AgglomerativeClustering.lvclass"(reference=w468, error in=w467, "accessors:R/W params"=w476) -> (reference out=w473:refnum<class "AgglomerativeClustering.lvclass">, error out=w477:errorcluster)
        n246 = call-dynamic "set_params.vi"("error in (no error)"=w477, "AgglomerativeClustering.lvclass 2"=w473) -> ("error out"=w461:errorcluster, "AgglomerativeClustering.lvclass"=w462:refnum<class "AgglomerativeClustering.lvclass">)  [unwired: 8 in]
        n247 = property class="AgglomerativeClustering.lvclass"(reference=w462, error in=w461, "accessors:R/W X"=w433) -> (reference out=w463:refnum<class "AgglomerativeClustering.lvclass">, error out=w478:errorcluster)
        n248 = call-dynamic "fit.vi"("error in (no error)"=w478, "AgglomerativeClustering.lvclass 2"=w463) -> ("error out"=w479:errorcluster, "AgglomerativeClustering.lvclass"=w464:refnum<class "AgglomerativeClustering.lvclass">)  [unwired: 8 in]
        n249 = call-dynamic "get_attributes.vi"("error in (no error)"=w479, "AgglomerativeClustering.lvclass 2"=w464) -> ("error out"=w480:errorcluster, "AgglomerativeClustering.lvclass"=w465:refnum<class "AgglomerativeClustering.lvclass">)  [unwired: 8 in]
        n250 = property class="AgglomerativeClustering.lvclass"(reference=w465, error in=w480) -> (reference out=w466:refnum<class "AgglomerativeClustering.lvclass">, error out=w475:errorcluster, "accessors:R/W attributes"=w458:T10)
        n251 = call-dynamic "closeSession.vi"("error in"=w475, "Python en entrée"=w466) -> ("error out"=w472:errorcluster)  [unwired: 8 in, 1 out]
        n252 = Unbundle By Name(w524) -> ("labels_"=w537:dbl[])
        n253 = Unbundle By Name(w502) -> ("labels_"=w503:dbl[])
        n254 = Unbundle By Name(w487) -> ("labels_"=w485:dbl[])
        n255 = Unbundle By Name(w458) -> ("labels_"=w460:dbl[])
        n256 = Build Array(w537) -> (w519:dbl[][])
        n257 = Build Array(w503) -> (w504:dbl[][])
        n258 = Build Array(w485) -> (w486:dbl[][])
        n259 = Build Array(w460) -> (w459:dbl[][])
        n260 = Transpose 2D Array(2D array=w519) -> (transposed array=w518:dbl[][])
        n261 = Transpose 2D Array(2D array=w504) -> (transposed array=w498:dbl[][])
        n262 = Transpose 2D Array(2D array=w486) -> (transposed array=w481:dbl[][])
        n263 = Transpose 2D Array(2D array=w459) -> (transposed array=w454:dbl[][])
        n264 = control-ref of="Plot 16"() -> (w523:refnum<vi>)
        n265 = Bundle By Name(cluster=T4 {"Plot"=refnum, "Data"={"X"=[], "Predict"=[]}, "Indexe"={"X"=0, "Y"=1}, "Point Property"={"Style"=enum."Full circle", "Label Color"=[8978528, 4367871, 1985280]}} ("Parameters"), "Plot"=w523, "Data.X"=w433, "Data.Predict"=w518, "Indexe"=cluster{"X":i32, "Y":i32} {"X"=0, "Y"=1}, "Point Property"=cluster{"Style":T3, "Label Color":u32[]} {"Style"=enum."Full circle", "Label Color"=[3381759, 15694592, 51218]}) -> (w522:T4)
        n266 = control-ref of="Plot 15"() -> (w500:refnum<vi>)
        n267 = control-ref of="Plot 14"() -> (w484:refnum<vi>)
        n268 = Bundle By Name(cluster=T4 {"Plot"=refnum, "Data"={"X"=[], "Predict"=[]}, "Indexe"={"X"=0, "Y"=1}, "Point Property"={"Style"=enum."Full circle", "Label Color"=[8978528, 4367871, 1985280]}} ("Parameters"), "Plot"=w500, "Data.X"=w433, "Data.Predict"=w498, "Indexe"=cluster{"X":i32, "Y":i32} {"X"=0, "Y"=1}, "Point Property"=cluster{"Style":T3, "Label Color":u32[]} {"Style"=enum."Full circle", "Label Color"=[3381759, 15694592, 51218]}) -> (w501:T4)
        n269 = control-ref of="Plot 13"() -> (w456:refnum<vi>)
        n270 = call "2DPredictedClassification.vi"("error in"=w472, "Parameters"=w522) -> ("error out"=w499:errorcluster)  [unwired: 9 in]
        n271 = Bundle By Name(cluster=T4 {"Plot"=refnum, "Data"={"X"=[], "Predict"=[]}, "Indexe"={"X"=0, "Y"=1}, "Point Property"={"Style"=enum."Full circle", "Label Color"=[8978528, 4367871, 1985280]}} ("Parameters"), "Plot"=w484, "Data.X"=w433, "Data.Predict"=w481, "Indexe"=cluster{"X":i32, "Y":i32} {"X"=0, "Y"=1}, "Point Property"=cluster{"Style":T3, "Label Color":u32[]} {"Style"=enum."Full circle", "Label Color"=[3381759, 15694592, 51218]}) -> (w483:T4)
        n272 = Bundle By Name(cluster=T4 {"Plot"=refnum, "Data"={"X"=[], "Predict"=[]}, "Indexe"={"X"=0, "Y"=1}, "Point Property"={"Style"=enum."Full circle", "Label Color"=[8978528, 4367871, 1985280]}} ("Parameters"), "Plot"=w456, "Data.X"=w433, "Data.Predict"=w454, "Indexe"=cluster{"X":i32, "Y":i32} {"X"=0, "Y"=1}, "Point Property"=cluster{"Style":T3, "Label Color":u32[]} {"Style"=enum."Full circle", "Label Color"=[3381759, 15694592, 51218]}) -> (w457:T4)
        n273 = call "2DPredictedClassification.vi"("error in"=w499, "Parameters"=w501) -> ("error out"=w482:errorcluster)  [unwired: 9 in]
        n274 = call "2DPredictedClassification.vi"("error in"=w482, "Parameters"=w483) -> ("error out"=w455:errorcluster)  [unwired: 9 in]
        n275 = call "2DPredictedClassification.vi"("error in"=w455, "Parameters"=w457) -> ("error out"=w435:errorcluster)  [unwired: 9 in]
      }
      frame 8 {
        # "Generate blobs with varied variances datasets and normalize dataset for easier parameter selection."
        n276 = Bundle By Name(cluster=T8 {"n_samples"=[100], "n_features"=2, "centers"=[], "cluster_std"=[1.0], "centermin"=-10.0, "centermax"=10.0, "shuffle"=TRUE, "random_state"=-1, "Returns"="X"} ("make_blobs"), "n_samples"=i32[] [1500], "random_state"=170, "cluster_std"=dbl[] [1.0, 2.5, 0.5]) -> (w549:T8)
        n277 = call "Blobs.vi"("error in (no error)"=w540, "make_blobs"=w549) -> ("error out"=w559:errorcluster, "Data"=w548:T9)  [unwired: 8 in]
        n278 = Unbundle By Name(w548) -> ("2DArray"=w558:string[][])
        n279 = call-poly "Processing Data.vi"("error in (no error)"=w559) -> ("error out"=w551:errorcluster, "StandardScaler.lvclass"=w550:refnum<class "StandardScaler.lvclass">)  [unwired: 9 in]
        n280 = call-dynamic "Fit Transform.vi"("Type X"=T1."Numeric Array", "error in (no error)"=w551, "X"=w558, "StandardScaler.lvclass"=w550) -> ("error out"=w553:errorcluster, "Data"=w554:T9, "StandardScaler.lvclass"=w552:refnum<class "StandardScaler.lvclass">)  [unwired: 5 in]
        n281 = Unbundle By Name(w554) -> ("2DArray"=w556:string[][])
        n282 = call-dynamic "ClosePython.vi"("error in (no error)"=w553, "Scikit-learn en entrée"=w552) -> ("error out"=w557:errorcluster)  [unwired: 8 in, 1 out]
        n283 = call "ArrayCharToString.vi"("TAB"=w556) -> ("Instruction"=w555:string)  [unwired: 10 in]
        n284 = call "StringToArrayFloat.vi"("entrée d'erreur (pas d'erreur)"=w557, "Return value"=w555) -> ("error IO"=w542:errorcluster, "2DArray"=w539:dbl[][])  [unwired: 7 in, 1 out]
        "varied" <- w539
      }
      frame 9 {
        # "Realize different linkage methods for hierarchical clustering on blobs with varied variances datasets."
        n285 = call-poly "Unsupervised.vi"("error in"=w561) -> ("error out"=w588:errorcluster, "out"=w587:refnum<class "AgglomerativeClustering.lvclass">)  [unwired: 9 in]
        n286 = Bundle By Name(cluster=T5 {"n_clusters"={"n_clusters_type"="int", "n_clusters_int"=0.0}, "affinity"={"affinity_type"="euclidean", "affinity_function"="metric_function"}, "memory"="", "connectivity"={"connectivity_type"="None", "connectivity_list"=[]}, "compute_full_tree"={"compute_full_tree_type"="auto", "compute_full_tree_bool"=FALSE}, "linkage"="ward", "distance_threshold"={"distance_threshold_type"="None", "distance_threshold_float"=0.0}, "compute_distances"=FALSE} ("output cluster"), "n_clusters"=T6 {"n_clusters_type"="int", "n_clusters_int"=3.0}, "linkage"="ward") -> (w611:T5)
        n287 = Bundle By Name(cluster=w611, "linkage"="complete") -> (w626:T5)
        n288 = call-dynamic "init.vi"("error in (no error)"=w588, "Model en entrée"=w587) -> ("error out"=w589:errorcluster, "Model en sortie"=w583:refnum<class "AgglomerativeClustering.lvclass">)  [unwired: 8 in]
        n289 = Bundle By Name(cluster=w626, "linkage"="average") -> (w644:T5)
        n290 = Bundle By Name(cluster=w644, "linkage"="single") -> (w642:T5)
        n291 = property class="AgglomerativeClustering.lvclass"(reference=w583, error in=w589, "accessors:R/W params"=w611) -> (reference out=w584:refnum<class "AgglomerativeClustering.lvclass">, error out=w590:errorcluster)
        n292 = call-dynamic "set_params.vi"("error in (no error)"=w590, "AgglomerativeClustering.lvclass 2"=w584) -> ("error out"=w591:errorcluster, "AgglomerativeClustering.lvclass"=w585:refnum<class "AgglomerativeClustering.lvclass">)  [unwired: 8 in]
        n293 = property class="AgglomerativeClustering.lvclass"(reference=w585, error in=w591, "accessors:R/W X"=w560) -> (reference out=w582:refnum<class "AgglomerativeClustering.lvclass">, error out=w592:errorcluster)
        n294 = call-dynamic "fit.vi"("error in (no error)"=w592, "AgglomerativeClustering.lvclass 2"=w582) -> ("error out"=w593:errorcluster, "AgglomerativeClustering.lvclass"=w586:refnum<class "AgglomerativeClustering.lvclass">)  [unwired: 8 in]
        n295 = call-dynamic "get_attributes.vi"("error in (no error)"=w593, "AgglomerativeClustering.lvclass 2"=w586) -> ("error out"=w598:errorcluster, "AgglomerativeClustering.lvclass"=w597:refnum<class "AgglomerativeClustering.lvclass">)  [unwired: 8 in]
        n296 = property class="AgglomerativeClustering.lvclass"(reference=w597, error in=w598) -> (reference out=w612:refnum<class "AgglomerativeClustering.lvclass">, error out=w613:errorcluster, "accessors:R/W attributes"=w594:T10)
        n297 = property class="AgglomerativeClustering.lvclass"(reference=w612, error in=w613, "accessors:R/W params"=w626) -> (reference out=w609:refnum<class "AgglomerativeClustering.lvclass">, error out=w606:errorcluster)
        n298 = call-dynamic "set_params.vi"("error in (no error)"=w606, "AgglomerativeClustering.lvclass 2"=w609) -> ("error out"=w605:errorcluster, "AgglomerativeClustering.lvclass"=w608:refnum<class "AgglomerativeClustering.lvclass">)  [unwired: 8 in]
        n299 = property class="AgglomerativeClustering.lvclass"(reference=w608, error in=w605, "accessors:R/W X"=w560) -> (reference out=w610:refnum<class "AgglomerativeClustering.lvclass">, error out=w604:errorcluster)
        n300 = call-dynamic "fit.vi"("error in (no error)"=w604, "AgglomerativeClustering.lvclass 2"=w610) -> ("error out"=w603:errorcluster, "AgglomerativeClustering.lvclass"=w607:refnum<class "AgglomerativeClustering.lvclass">)  [unwired: 8 in]
        n301 = call-dynamic "get_attributes.vi"("error in (no error)"=w603, "AgglomerativeClustering.lvclass 2"=w607) -> ("error out"=w601:errorcluster, "AgglomerativeClustering.lvclass"=w602:refnum<class "AgglomerativeClustering.lvclass">)  [unwired: 8 in]
        n302 = property class="AgglomerativeClustering.lvclass"(reference=w602, error in=w601) -> (reference out=w627:refnum<class "AgglomerativeClustering.lvclass">, error out=w628:errorcluster, "accessors:R/W attributes"=w616:T10)
        n303 = property class="AgglomerativeClustering.lvclass"(reference=w627, error in=w628, "accessors:R/W params"=w644) -> (reference out=w629:refnum<class "AgglomerativeClustering.lvclass">, error out=w621:errorcluster)
        n304 = call-dynamic "set_params.vi"("error in (no error)"=w621, "AgglomerativeClustering.lvclass 2"=w629) -> ("error out"=w622:errorcluster, "AgglomerativeClustering.lvclass"=w630:refnum<class "AgglomerativeClustering.lvclass">)  [unwired: 8 in]
        n305 = property class="AgglomerativeClustering.lvclass"(reference=w630, error in=w622, "accessors:R/W X"=w560) -> (reference out=w647:refnum<class "AgglomerativeClustering.lvclass">, error out=w623:errorcluster)
        n306 = call-dynamic "fit.vi"("error in (no error)"=w623, "AgglomerativeClustering.lvclass 2"=w647) -> ("error out"=w624:errorcluster, "AgglomerativeClustering.lvclass"=w648:refnum<class "AgglomerativeClustering.lvclass">)  [unwired: 8 in]
        n307 = call-dynamic "get_attributes.vi"("error in (no error)"=w624, "AgglomerativeClustering.lvclass 2"=w648) -> ("error out"=w625:errorcluster, "AgglomerativeClustering.lvclass"=w649:refnum<class "AgglomerativeClustering.lvclass">)  [unwired: 8 in]
        n308 = property class="AgglomerativeClustering.lvclass"(reference=w649, error in=w625) -> (reference out=w650:refnum<class "AgglomerativeClustering.lvclass">, error out=w651:errorcluster, "accessors:R/W attributes"=w631:T10)
        n309 = property class="AgglomerativeClustering.lvclass"(reference=w650, error in=w651, "accessors:R/W params"=w642) -> (reference out=w645:refnum<class "AgglomerativeClustering.lvclass">, error out=w641:errorcluster)
        n310 = call-dynamic "set_params.vi"("error in (no error)"=w641, "AgglomerativeClustering.lvclass 2"=w645) -> ("error out"=w657:errorcluster, "AgglomerativeClustering.lvclass"=w656:refnum<class "AgglomerativeClustering.lvclass">)  [unwired: 8 in]
        n311 = property class="AgglomerativeClustering.lvclass"(reference=w656, error in=w657, "accessors:R/W X"=w560) -> (reference out=w655:refnum<class "AgglomerativeClustering.lvclass">, error out=w640:errorcluster)
        n312 = call-dynamic "fit.vi"("error in (no error)"=w640, "AgglomerativeClustering.lvclass 2"=w655) -> ("error out"=w639:errorcluster, "AgglomerativeClustering.lvclass"=w654:refnum<class "AgglomerativeClustering.lvclass">)  [unwired: 8 in]
        n313 = call-dynamic "get_attributes.vi"("error in (no error)"=w639, "AgglomerativeClustering.lvclass 2"=w654) -> ("error out"=w638:errorcluster, "AgglomerativeClustering.lvclass"=w653:refnum<class "AgglomerativeClustering.lvclass">)  [unwired: 8 in]
        n314 = property class="AgglomerativeClustering.lvclass"(reference=w653, error in=w638) -> (reference out=w652:refnum<class "AgglomerativeClustering.lvclass">, error out=w643:errorcluster, "accessors:R/W attributes"=w660:T10)
        n315 = call-dynamic "closeSession.vi"("error in"=w643, "Python en entrée"=w652) -> ("error out"=w646:errorcluster)  [unwired: 8 in, 1 out]
        n316 = Unbundle By Name(w594) -> ("labels_"=w581:dbl[])
        n317 = Unbundle By Name(w616) -> ("labels_"=w615:dbl[])
        n318 = Unbundle By Name(w660) -> ("labels_"=w658:dbl[])
        n319 = Unbundle By Name(w631) -> ("labels_"=w633:dbl[])
        n320 = Build Array(w581) -> (w599:dbl[][])
        n321 = Build Array(w615) -> (w614:dbl[][])
        n322 = Build Array(w658) -> (w659:dbl[][])
        n323 = Build Array(w633) -> (w632:dbl[][])
        n324 = Transpose 2D Array(2D array=w599) -> (transposed array=w600:dbl[][])
        n325 = Transpose 2D Array(2D array=w614) -> (transposed array=w620:dbl[][])
        n326 = Transpose 2D Array(2D array=w659) -> (transposed array=w664:dbl[][])
        n327 = Transpose 2D Array(2D array=w632) -> (transposed array=w637:dbl[][])
        n328 = control-ref of="Plot 20"() -> (w595:refnum<vi>)
        n329 = Bundle By Name(cluster=T4 {"Plot"=refnum, "Data"={"X"=[], "Predict"=[]}, "Indexe"={"X"=0, "Y"=1}, "Point Property"={"Style"=enum."Full circle", "Label Color"=[8978528, 4367871, 1985280]}} ("Parameters"), "Plot"=w595, "Data.X"=w560, "Data.Predict"=w600, "Indexe"=cluster{"X":i32, "Y":i32} {"X"=0, "Y"=1}, "Point Property"=cluster{"Style":T3, "Label Color":u32[]} {"Style"=enum."Full circle", "Label Color"=[3381759, 15694592, 51218]}) -> (w596:T4)
        n330 = control-ref of="Plot 19"() -> (w618:refnum<vi>)
        n331 = control-ref of="Plot 18"() -> (w634:refnum<vi>)
        n332 = Bundle By Name(cluster=T4 {"Plot"=refnum, "Data"={"X"=[], "Predict"=[]}, "Indexe"={"X"=0, "Y"=1}, "Point Property"={"Style"=enum."Full circle", "Label Color"=[8978528, 4367871, 1985280]}} ("Parameters"), "Plot"=w618, "Data.X"=w560, "Data.Predict"=w620, "Indexe"=cluster{"X":i32, "Y":i32} {"X"=0, "Y"=1}, "Point Property"=cluster{"Style":T3, "Label Color":u32[]} {"Style"=enum."Full circle", "Label Color"=[3381759, 15694592, 51218]}) -> (w617:T4)
        n333 = control-ref of="Plot 17"() -> (w662:refnum<vi>)
        n334 = call "2DPredictedClassification.vi"("error in"=w646, "Parameters"=w596) -> ("error out"=w619:errorcluster)  [unwired: 9 in]
        n335 = Bundle By Name(cluster=T4 {"Plot"=refnum, "Data"={"X"=[], "Predict"=[]}, "Indexe"={"X"=0, "Y"=1}, "Point Property"={"Style"=enum."Full circle", "Label Color"=[8978528, 4367871, 1985280]}} ("Parameters"), "Plot"=w634, "Data.X"=w560, "Data.Predict"=w637, "Indexe"=cluster{"X":i32, "Y":i32} {"X"=0, "Y"=1}, "Point Property"=cluster{"Style":T3, "Label Color":u32[]} {"Style"=enum."Full circle", "Label Color"=[3381759, 15694592, 51218]}) -> (w635:T4)
        n336 = Bundle By Name(cluster=T4 {"Plot"=refnum, "Data"={"X"=[], "Predict"=[]}, "Indexe"={"X"=0, "Y"=1}, "Point Property"={"Style"=enum."Full circle", "Label Color"=[8978528, 4367871, 1985280]}} ("Parameters"), "Plot"=w662, "Data.X"=w560, "Data.Predict"=w664, "Indexe"=cluster{"X":i32, "Y":i32} {"X"=0, "Y"=1}, "Point Property"=cluster{"Style":T3, "Label Color":u32[]} {"Style"=enum."Full circle", "Label Color"=[3381759, 15694592, 51218]}) -> (w661:T4)
        n337 = call "2DPredictedClassification.vi"("error in"=w619, "Parameters"=w617) -> ("error out"=w636:errorcluster)  [unwired: 9 in]
        n338 = call "2DPredictedClassification.vi"("error in"=w636, "Parameters"=w635) -> ("error out"=w663:errorcluster)  [unwired: 9 in]
        n339 = call "2DPredictedClassification.vi"("error in"=w663, "Parameters"=w661) -> ("error out"=w562:errorcluster)  [unwired: 9 in]
      }
      frame 10 {
        # "Generate random datasets and normalize dataset for easier parameter selection."
        n340 = for {
          N: 2 -> [_]
          tunnel: dbl[] [] ("2DArray") -> [w685]
          tunnel: [w686] -> w674 mode=indexing
          n341 = for {
            N: 1500 -> [_]
            shift-right: [w689] -> w686
            shift-left: w685 -> [w688]
            n342 = Random Number (0-1)() -> (number: 0 to 1=w687:dbl)
            n343 = Insert Into Array(array=w688, new element=w687) -> (w689:dbl[])  [unwired: 1 in]
          }
        }
        n344 = Transpose 2D Array(2D array=w674) -> (transposed array=w683:dbl[][])
        n345 = call-poly "Processing Data.vi"("error in (no error)"=w667) -> ("error out"=w681:errorcluster, "StandardScaler.lvclass"=w682:refnum<class "StandardScaler.lvclass">)  [unwired: 9 in]
        n346 = call "ArrayFloatToString.vi"("2D Data"=w683) -> ("Array"=w670:string[][])  [unwired: 9 in, 1 out]
        n347 = call-dynamic "Fit Transform.vi"("Type X"=T1."Numeric Array", "error in (no error)"=w681, "X"=w670, "StandardScaler.lvclass"=w682) -> ("error out"=w679:errorcluster, "Data"=w678:T9, "StandardScaler.lvclass"=w680:refnum<class "StandardScaler.lvclass">)  [unwired: 5 in]
        n348 = Unbundle By Name(w678) -> ("2DArray"=w676:string[][])
        n349 = call-dynamic "ClosePython.vi"("error in (no error)"=w679, "Scikit-learn en entrée"=w680) -> ("error out"=w675:errorcluster)  [unwired: 8 in, 1 out]
        n350 = call "ArrayCharToString.vi"("TAB"=w676) -> ("Instruction"=w677:string)  [unwired: 10 in]
        n351 = call "StringToArrayFloat.vi"("entrée d'erreur (pas d'erreur)"=w675, "Return value"=w677) -> ("error IO"=w669:errorcluster, "2DArray"=w666:dbl[][])  [unwired: 7 in, 1 out]
        "no_structure" <- w666
      }
      frame 11 {
        # "Realize different linkage methods for hierarchical clustering on random datasets."
        n352 = Bundle By Name(cluster=T5 {"n_clusters"={"n_clusters_type"="int", "n_clusters_int"=0.0}, "affinity"={"affinity_type"="euclidean", "affinity_function"="metric_function"}, "memory"="", "connectivity"={"connectivity_type"="None", "connectivity_list"=[]}, "compute_full_tree"={"compute_full_tree_type"="auto", "compute_full_tree_bool"=FALSE}, "linkage"="ward", "distance_threshold"={"distance_threshold_type"="None", "distance_threshold_float"=0.0}, "compute_distances"=FALSE} ("output cluster"), "n_clusters"=T6 {"n_clusters_type"="int", "n_clusters_int"=3.0}, "linkage"="ward") -> (w764:T5)
        n353 = call-poly "Unsupervised.vi"("error in"=w691) -> ("error out"=w787:errorcluster, "out"=w788:refnum<class "AgglomerativeClustering.lvclass">)  [unwired: 9 in]
        n354 = Bundle By Name(cluster=w764, "linkage"="complete") -> (w749:T5)
        n355 = Bundle By Name(cluster=w749, "linkage"="average") -> (w731:T5)
        n356 = call-dynamic "init.vi"("error in (no error)"=w787, "Model en entrée"=w788) -> ("error out"=w786:errorcluster, "Model en sortie"=w792:refnum<class "AgglomerativeClustering.lvclass">)  [unwired: 8 in]
        n357 = Bundle By Name(cluster=w731, "linkage"="single") -> (w733:T5)
        n358 = property class="AgglomerativeClustering.lvclass"(reference=w792, error in=w786, "accessors:R/W params"=w764) -> (reference out=w791:refnum<class "AgglomerativeClustering.lvclass">, error out=w785:errorcluster)
        n359 = call-dynamic "set_params.vi"("error in (no error)"=w785, "AgglomerativeClustering.lvclass 2"=w791) -> ("error out"=w784:errorcluster, "AgglomerativeClustering.lvclass"=w790:refnum<class "AgglomerativeClustering.lvclass">)  [unwired: 8 in]
        n360 = property class="AgglomerativeClustering.lvclass"(reference=w790, error in=w784, "accessors:R/W X"=w690) -> (reference out=w793:refnum<class "AgglomerativeClustering.lvclass">, error out=w783:errorcluster)
        n361 = call-dynamic "fit.vi"("error in (no error)"=w783, "AgglomerativeClustering.lvclass 2"=w793) -> ("error out"=w782:errorcluster, "AgglomerativeClustering.lvclass"=w789:refnum<class "AgglomerativeClustering.lvclass">)  [unwired: 8 in]
        n362 = call-dynamic "get_attributes.vi"("error in (no error)"=w782, "AgglomerativeClustering.lvclass 2"=w789) -> ("error out"=w777:errorcluster, "AgglomerativeClustering.lvclass"=w778:refnum<class "AgglomerativeClustering.lvclass">)  [unwired: 8 in]
        n363 = property class="AgglomerativeClustering.lvclass"(reference=w778, error in=w777) -> (reference out=w763:refnum<class "AgglomerativeClustering.lvclass">, error out=w762:errorcluster, "accessors:R/W attributes"=w781:T10)
        n364 = property class="AgglomerativeClustering.lvclass"(reference=w763, error in=w762, "accessors:R/W params"=w749) -> (reference out=w766:refnum<class "AgglomerativeClustering.lvclass">, error out=w769:errorcluster)
        n365 = call-dynamic "set_params.vi"("error in (no error)"=w769, "AgglomerativeClustering.lvclass 2"=w766) -> ("error out"=w770:errorcluster, "AgglomerativeClustering.lvclass"=w767:refnum<class "AgglomerativeClustering.lvclass">)  [unwired: 8 in]
        n366 = property class="AgglomerativeClustering.lvclass"(reference=w767, error in=w770, "accessors:R/W X"=w690) -> (reference out=w765:refnum<class "AgglomerativeClustering.lvclass">, error out=w771:errorcluster)
        n367 = call-dynamic "fit.vi"("error in (no error)"=w771, "AgglomerativeClustering.lvclass 2"=w765) -> ("error out"=w772:errorcluster, "AgglomerativeClustering.lvclass"=w768:refnum<class "AgglomerativeClustering.lvclass">)  [unwired: 8 in]
        n368 = call-dynamic "get_attributes.vi"("error in (no error)"=w772, "AgglomerativeClustering.lvclass 2"=w768) -> ("error out"=w774:errorcluster, "AgglomerativeClustering.lvclass"=w773:refnum<class "AgglomerativeClustering.lvclass">)  [unwired: 8 in]
        n369 = property class="AgglomerativeClustering.lvclass"(reference=w773, error in=w774) -> (reference out=w748:refnum<class "AgglomerativeClustering.lvclass">, error out=w747:errorcluster, "accessors:R/W attributes"=w759:T10)
        n370 = property class="AgglomerativeClustering.lvclass"(reference=w748, error in=w747, "accessors:R/W params"=w731) -> (reference out=w746:refnum<class "AgglomerativeClustering.lvclass">, error out=w754:errorcluster)
        n371 = call-dynamic "set_params.vi"("error in (no error)"=w754, "AgglomerativeClustering.lvclass 2"=w746) -> ("error out"=w753:errorcluster, "AgglomerativeClustering.lvclass"=w745:refnum<class "AgglomerativeClustering.lvclass">)  [unwired: 8 in]
        n372 = property class="AgglomerativeClustering.lvclass"(reference=w745, error in=w753, "accessors:R/W X"=w690) -> (reference out=w728:refnum<class "AgglomerativeClustering.lvclass">, error out=w752:errorcluster)
        n373 = call-dynamic "fit.vi"("error in (no error)"=w752, "AgglomerativeClustering.lvclass 2"=w728) -> ("error out"=w751:errorcluster, "AgglomerativeClustering.lvclass"=w727:refnum<class "AgglomerativeClustering.lvclass">)  [unwired: 8 in]
        n374 = call-dynamic "get_attributes.vi"("error in (no error)"=w751, "AgglomerativeClustering.lvclass 2"=w727) -> ("error out"=w750:errorcluster, "AgglomerativeClustering.lvclass"=w726:refnum<class "AgglomerativeClustering.lvclass">)  [unwired: 8 in]
        n375 = property class="AgglomerativeClustering.lvclass"(reference=w726, error in=w750) -> (reference out=w725:refnum<class "AgglomerativeClustering.lvclass">, error out=w724:errorcluster, "accessors:R/W attributes"=w744:T10)
        n376 = property class="AgglomerativeClustering.lvclass"(reference=w725, error in=w724, "accessors:R/W params"=w733) -> (reference out=w730:refnum<class "AgglomerativeClustering.lvclass">, error out=w734:errorcluster)
        n377 = call-dynamic "set_params.vi"("error in (no error)"=w734, "AgglomerativeClustering.lvclass 2"=w730) -> ("error out"=w718:errorcluster, "AgglomerativeClustering.lvclass"=w719:refnum<class "AgglomerativeClustering.lvclass">)  [unwired: 8 in]
        n378 = property class="AgglomerativeClustering.lvclass"(reference=w719, error in=w718, "accessors:R/W X"=w690) -> (reference out=w720:refnum<class "AgglomerativeClustering.lvclass">, error out=w735:errorcluster)
        n379 = call-dynamic "fit.vi"("error in (no error)"=w735, "AgglomerativeClustering.lvclass 2"=w720) -> ("error out"=w736:errorcluster, "AgglomerativeClustering.lvclass"=w721:refnum<class "AgglomerativeClustering.lvclass">)  [unwired: 8 in]
        n380 = call-dynamic "get_attributes.vi"("error in (no error)"=w736, "AgglomerativeClustering.lvclass 2"=w721) -> ("error out"=w737:errorcluster, "AgglomerativeClustering.lvclass"=w722:refnum<class "AgglomerativeClustering.lvclass">)  [unwired: 8 in]
        n381 = property class="AgglomerativeClustering.lvclass"(reference=w722, error in=w737) -> (reference out=w723:refnum<class "AgglomerativeClustering.lvclass">, error out=w732:errorcluster, "accessors:R/W attributes"=w715:T10)
        n382 = call-dynamic "closeSession.vi"("error in"=w732, "Python en entrée"=w723) -> ("error out"=w729:errorcluster)  [unwired: 8 in, 1 out]
        n383 = Unbundle By Name(w744) -> ("labels_"=w742:dbl[])
        n384 = Unbundle By Name(w759) -> ("labels_"=w760:dbl[])
        n385 = Unbundle By Name(w715) -> ("labels_"=w717:dbl[])
        n386 = Unbundle By Name(w781) -> ("labels_"=w794:dbl[])
        n387 = Build Array(w742) -> (w743:dbl[][])
        n388 = Build Array(w794) -> (w776:dbl[][])
        n389 = Build Array(w760) -> (w761:dbl[][])
        n390 = Build Array(w717) -> (w716:dbl[][])
        n391 = Transpose 2D Array(2D array=w743) -> (transposed array=w738:dbl[][])
        n392 = Transpose 2D Array(2D array=w761) -> (transposed array=w755:dbl[][])
        n393 = Transpose 2D Array(2D array=w716) -> (transposed array=w711:dbl[][])
        n394 = Transpose 2D Array(2D array=w776) -> (transposed array=w775:dbl[][])
        n395 = control-ref of="Plot 24"() -> (w780:refnum<vi>)
        n396 = Bundle By Name(cluster=T4 {"Plot"=refnum, "Data"={"X"=[], "Predict"=[]}, "Indexe"={"X"=0, "Y"=1}, "Point Property"={"Style"=enum."Full circle", "Label Color"=[8978528, 4367871, 1985280]}} ("Parameters"), "Plot"=w780, "Data.X"=w690, "Data.Predict"=w775, "Indexe"=cluster{"X":i32, "Y":i32} {"X"=0, "Y"=1}, "Point Property"=cluster{"Style":T3, "Label Color":u32[]} {"Style"=enum."Full circle", "Label Color"=[3381759, 15694592, 51218]}) -> (w779:T4)
        n397 = control-ref of="Plot 23"() -> (w757:refnum<vi>)
        n398 = control-ref of="Plot 22"() -> (w741:refnum<vi>)
        n399 = Bundle By Name(cluster=T4 {"Plot"=refnum, "Data"={"X"=[], "Predict"=[]}, "Indexe"={"X"=0, "Y"=1}, "Point Property"={"Style"=enum."Full circle", "Label Color"=[8978528, 4367871, 1985280]}} ("Parameters"), "Plot"=w757, "Data.X"=w690, "Data.Predict"=w755, "Indexe"=cluster{"X":i32, "Y":i32} {"X"=0, "Y"=1}, "Point Property"=cluster{"Style":T3, "Label Color":u32[]} {"Style"=enum."Full circle", "Label Color"=[3381759, 15694592, 51218]}) -> (w758:T4)
        n400 = control-ref of="Plot 21"() -> (w713:refnum<vi>)
        n401 = call "2DPredictedClassification.vi"("error in"=w729, "Parameters"=w779) -> ("error out"=w756:errorcluster)  [unwired: 9 in]
        n402 = Bundle By Name(cluster=T4 {"Plot"=refnum, "Data"={"X"=[], "Predict"=[]}, "Indexe"={"X"=0, "Y"=1}, "Point Property"={"Style"=enum."Full circle", "Label Color"=[8978528, 4367871, 1985280]}} ("Parameters"), "Plot"=w741, "Data.X"=w690, "Data.Predict"=w738, "Indexe"=cluster{"X":i32, "Y":i32} {"X"=0, "Y"=1}, "Point Property"=cluster{"Style":T3, "Label Color":u32[]} {"Style"=enum."Full circle", "Label Color"=[3381759, 15694592, 51218]}) -> (w740:T4)
        n403 = Bundle By Name(cluster=T4 {"Plot"=refnum, "Data"={"X"=[], "Predict"=[]}, "Indexe"={"X"=0, "Y"=1}, "Point Property"={"Style"=enum."Full circle", "Label Color"=[8978528, 4367871, 1985280]}} ("Parameters"), "Plot"=w713, "Data.X"=w690, "Data.Predict"=w711, "Indexe"=cluster{"X":i32, "Y":i32} {"X"=0, "Y"=1}, "Point Property"=cluster{"Style":T3, "Label Color":u32[]} {"Style"=enum."Full circle", "Label Color"=[3381759, 15694592, 51218]}) -> (w714:T4)
        n404 = call "2DPredictedClassification.vi"("error in"=w756, "Parameters"=w758) -> ("error out"=w739:errorcluster)  [unwired: 9 in]
        n405 = call "2DPredictedClassification.vi"("error in"=w739, "Parameters"=w740) -> ("error out"=w712:errorcluster)  [unwired: 9 in]
        n406 = call "2DPredictedClassification.vi"("error in"=w712, "Parameters"=w714) -> ("error out"=w693:errorcluster)  [unwired: 9 in]
      }
    }
  }
  "error out" <- w1
